vi "运维调试_氨氮.vi"() -> ()   [LabVIEW 2016, in "斯坦道氨氮.lvlib"]
uses:
  <vilib>/Utility/miscctls.llb/LVPointTypeDef.ctl
  <vilib>/Utility/config.llb/NI_LVConfig.lvlib
  <vilib>/ptbypt/NI_PtbyPt.lvlib
panel:
  in  "远程标样校准":enum16{"标液1", "标液2", "标液3", "标液4"}(ring)
  in  "远程校准量程":enum16{"低量程", "高量程"}(ring)
  in  "曲线模型 2":cluster{"X^2":dbl, "X":dbl, "B":dbl, "r^2":dbl}(xcontrol)
  out "固件版本号":string
  in  "定时设置":cluster{"启动":bool, "控制命令":T1, "测量参数":T2}(xcontrol)
  out "模块版本号":string
  in  "校准按钮":T3
  out "单位:":T4(ring)
  out "运行状态":T5 {"数据时间:" format="%<%y/%m/%d %H:%M:%S>T"; "仪器时间:" format="%<%y/%m/%d %H:%M:%S>T"}
  out "二级权限":bool
  out "一级权限":bool
  out "输入密码":u32
  out "布尔":bool
  in  "仪器参数设置":bool
  in  "流程固件":bool
  in  "量程参数读取写入":T6
  in  "模块启用":bool
  in  "串口设置":bool
  in  "公式一键写入":bool
  in  "流程路径":path=path "C:/Users/STD/Documents/斯坦道流程文件/流程.xml"
  in  "曲线模型":cluster{"X^2":dbl, "X":dbl, "B":dbl, "r^2":dbl}(xcontrol)
  out "字符串":string
  in  "质控参数设置":bool
  out "温度2":sgl
  out "温度1":sgl
  out "ADC":sgl
  in  "数组":string[](array[string])
  in  "量程切换阈值写入":bool
  in  "量程切换阈值读取":bool
  in  "参数下拉列表":enum16{"总磷", "总氮", "氨氮"}(ring)=enum."氨氮"
  in  "量程下拉列表":enum16{"低量程", "高量程"}(ring)
  in  "测量模式下拉列表":enum16{"水样测量", "零点核查", "跨度核查", "标样核查", "加标回收"}(ring)
  in  "公式":cluster{"X^2":dbl, "X":dbl, "b":dbl}
  in  "写公式":bool
  in  "读公式":bool
  in  "返回":bool
  in  "设置":bool
  out "集成报警信息":string
  in  "停止":bool
  in  "手动启动":bool
  in  "单步测试":bool
  out "F3":sgl format="%#.6f"
  out "F2":sgl format="%#.6f"
  out "F1":sgl format="%#.6f"
  out "F0":sgl format="%#.6f"
  out "多列列表框":i32(listbox)
  # "参数设置"
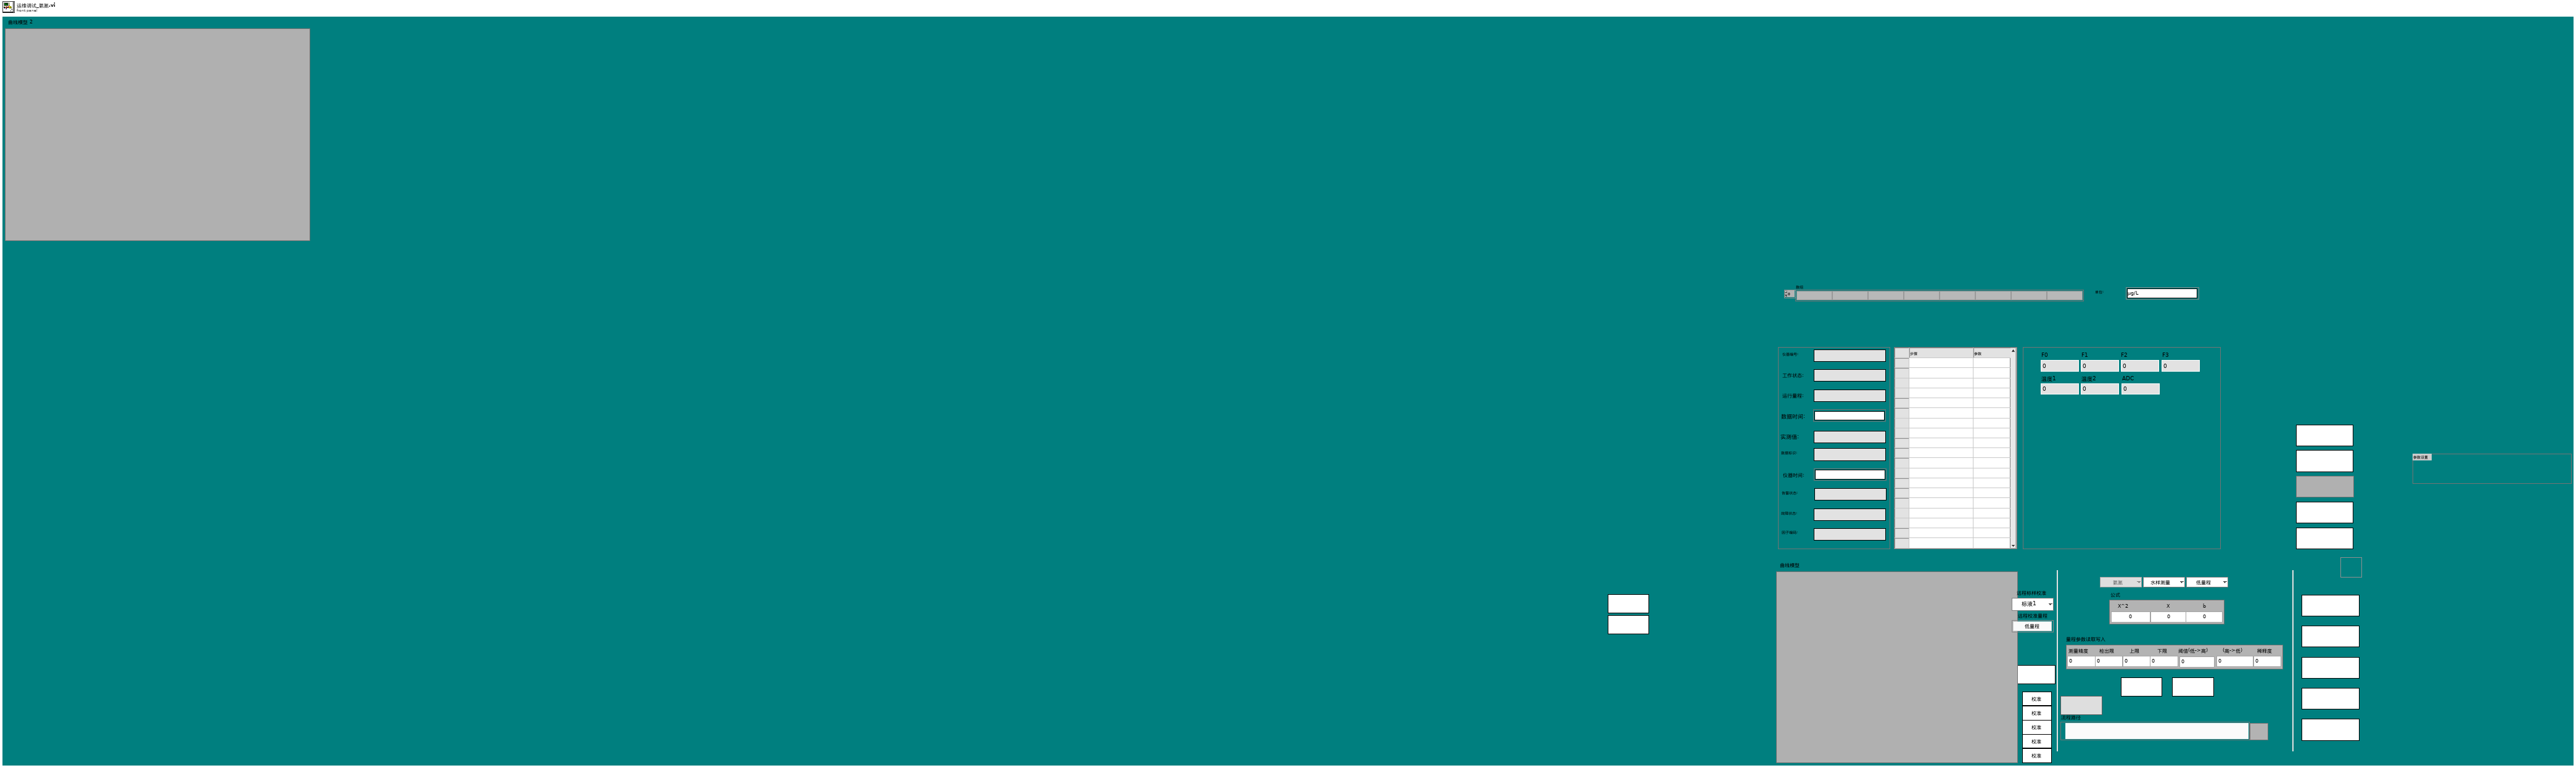
[diagram p1: front panel]
types:
  T1 = typedef "定时设置.xctl/国标控制命令.ctl" = enum16{"启动测量", "标样核查", "零点核查", "跨度核查", "空白测试", "平行样测试", "加标回收", "空白校准", "标样校准", "初始化（清洗）", "停止测试", "仪器重启", "校时", "模式设置", "测量间隔设置"}
  T2 = typedef "定时设置.xctl/测量参数.ctl" = u16
  T3 = cluster{"校准1":bool, "校准2":bool, "校准3":bool, "校准4":bool, "校准5":bool}
  T4 = enum16{"μg/L", "mg/L", "ppm", "mg/m3", "cm", "ppb", "μg/m3", "%", "nmol/mol", "μmol/mol", "MPN/L", "MPN/100ml", "ng/m3", "NTU", "无量纲", "mS/cm", "μS/cm", "℃", "mV", "cells/mL"}
  T5 = cluster{"仪器编号:":string, "工作状态:":string, "运行量程: ":string, "数据时间:":timestamp, "实测值:":string, "数据标识: ":string, "仪器时间:":timestamp, "告警状态: ":string, "故障状态:  ":string, "因子编码:":string}
  T6 = cluster{"测量精度":dbl, "检出限":dbl, "上限":dbl, "下限":dbl, "阈值(低->高)":dbl, "(高->低)":dbl, "稀释度":dbl}
  T7 = typedef "LVPointTypeDef.ctl" = cluster{"Horizontal":i16, "Vertical":i16}
  T8 = cluster{"时间源选择":enum16{"系统时间源", "仪器时间源"}, "外部时间源":timestamp}
  T9 = enum16{"空闲", "水样测试", "标样核查", "零点核查", "跨度核查", "空白测试", "平行样测试", "加标回收", "空白校准", "标样校准", "初始化（清洗）"}
  T10 = cluster{"系统时间":timestamp, "工作状态":enum16{"空闲", "水样测试", "标样核查", "零点核查", "跨度核查", "空白测试", "平行样测试", "加标回收", "空白校准", "标样校准", "初始化（清洗）"}, "测量模式":enum16{"待机", "连续模式", "周期模式", "定点模式", "受控模式", "手动模式"}, "告警代码":u16, "故障代码":u16, "日志代码":u16, "软件版本":u16, "F0":sgl, "F1":sgl, "F2":sgl, "F3":sgl, "T":sgl, "H":sgl, "id":u16, "flowid":u16, "量程":u16, "总磷控温温度1":sgl, "营养盐控温温度2":sgl, "ADC":sgl}
  T11 = enum32{"Bad", "Idle", "Run top level", "Running"}
  T12 = enum8{"Enabled", "Disabled", "Disabled and Grayed Out"}
  T13 = cluster{"运行模式":enum16{"维护模式", "常规模式", "应急模式", "质控模式"}, "质控频次":enum16{"关闭", "每天", "星期一", "星期二", "星期三", "星期四", "星期五", "星期六", "星期日"}, "空白核查时间":u16, "跨度核查时间":u16, "24H周期设置":bool[]}
  T14 = cluster{"因子编码":u32, "单位":u16, "标样参考值":sgl, "水样数据时间":timestamp, "水样实测值":sgl, "水样数据标识":string, "标样数据时间":timestamp, "标样实测值":sgl, "标样数据标识":string, "空白数据时间":timestamp, "空白实测值":sgl, "空白数据标识":string, "零点核查数据时间":timestamp, "零点核查实测值":sgl, "零点核查数据标识":string, "跨度核查数据时间":timestamp, "跨度核查实测值":sgl, "跨度核查数据标识":string, "加标回收数据时间":timestamp, "加标回收实测值":sgl, "加标回收数据标识":string, "平行样数据时间":timestamp, "平行样实测值":sgl, "平行样数据标识":string, "F0":sgl, "F1":sgl, "F2":sgl, "F3":sgl, "F4":sgl, "F5":sgl, "F6":sgl, "F7":sgl, "温度":sgl, "湿度":sgl, "X值":sgl, "fidrange":u16}
  T15 = cluster{"Major":u16, "Minor":u16, "Fix":u16, "Build":u16}
  T16 = typedef "NI_LVConfig.lvlib/Config Data RefNum.ctl" = refnum<k1>
  T17 = cluster{"时间标识":timestamp, "设备":string, "日志信息":string, "备注":string}
  T18 = cluster{"参数":string, "报警内容":string, "报警分析":string}
  T19 = cluster{"参数下拉列表":enum16{"总磷", "总氮", "氨氮"}, "测量模式下拉列表":enum16{"水样测量", "零点核查", "跨度核查", "标样核查", "加标回收"}, "量程下拉列表":enum16{"低量程", "高量程"}}
  T20 = cluster{"启动模式":enum16{"跨度核查", "水样测量", "空白核查", "标样核查", "加标回收"}, "启动参数":u16, "量程":enum16{"低量程", "高量程"}}
  T21 = cluster{"时间标识":timestamp, "设备":string, "日志信息":string, "流程参数":string}
  T22 = typedef "LVRowAndColumnUnsignedTypeDef.ctl" = cluster{"Row":u32, "Column":u32}
  T23 = cluster{"站号":u16, "量程切换":enum32{"H", "L", "AUTO"}, "控制命令":enum16{"启动测量", "标样核查", "零点核查", "跨度核查", "空白测试", "平行样测试", "加标回收", "空白校准", "标样校准", "初始化（清洗）", "停止测试", "仪器重启", "校时", "模式设置", "测量间隔设置"}, "模式设置":enum16{"待机", "连续模式", "周期模式", "定点模式", "受控模式", "手动模式"}, "测量间隔":u16}
  T24 = cluster{"标液浓度1":dbl, "标液浓度2":dbl, "标液浓度3":dbl, "标液浓度4":dbl, "标液浓度5":dbl}
  T25 = cluster{"水样测试量程模式":enum16{"H", "L", "AUTO"}, "空白核查量程模式":enum16{"H", "L", "AUTO"}, "跨度核查量程模式":enum16{"H", "L", "AUTO"}, "加标回收量程模式":enum16{"H", "L", "AUTO"}}
  T26 = cluster{"跨度值":dbl, "零点标准液浓度":dbl, "跨度标准液浓度":dbl, "标准液标准浓度":dbl}
  T27 = cluster{"确定":bool, "跨度值":dbl, "零点标准液浓度":dbl, "跨度标准液浓度":dbl, "标准液标准浓度":dbl}
  T28 = cluster{"测量量程":dbl, "测量精度":dbl, "测量间隔":dbl, "消解温度":dbl, "消解时长":dbl, "空白校准时间":timestamp, "曲线截距":dbl, "曲线斜率":dbl, "测量检出限":dbl, "测量信号值":dbl, "线性相关系数":dbl, "二次多项式系数":dbl, "标样校准时间":timestamp, "稀释倍数":dbl, "三项式系数":dbl, "空白标定系数":dbl, "量程系数":dbl, "F0/ORPA":dbl, "F1/ORPB":dbl, "F2/ORPK":dbl, "F3":dbl, "F4":dbl, "F5":dbl, "F6":dbl, "F7":dbl, "X0/滴定数":dbl, "量程":dbl}
  T29 = cluster{"确定":bool, "测量量程":dbl, "测量精度":dbl, "测量间隔":dbl, "消解温度":dbl, "消解时长":dbl, "空白校准时间":timestamp, "曲线截距":dbl, "曲线斜率":dbl, "测量检出限":dbl, "测量信号值":dbl, "线性相关系数":dbl, "二次多项式系数":dbl, "标样校准时间":timestamp, "稀释倍数":dbl, "三项式系数":dbl, "空白标定系数":dbl, "量程系数":dbl, "F0/ORPA":dbl, "F1/ORPB":dbl, "F2/ORPK":dbl, "F3":dbl, "F4":dbl, "F5":dbl, "F6":dbl, "F7":dbl, "X0/滴定数":dbl, "量程":dbl}
  T30 = cluster{"测量精度":u16, "检出限":dbl, "上限":dbl, "下限":dbl, "阈值（低->高）":dbl, "阈值（高->低）":dbl, "稀释度":dbl}
  T31 = enum16{"Left Button", "Center Button", "Right Button", "Window Close"}
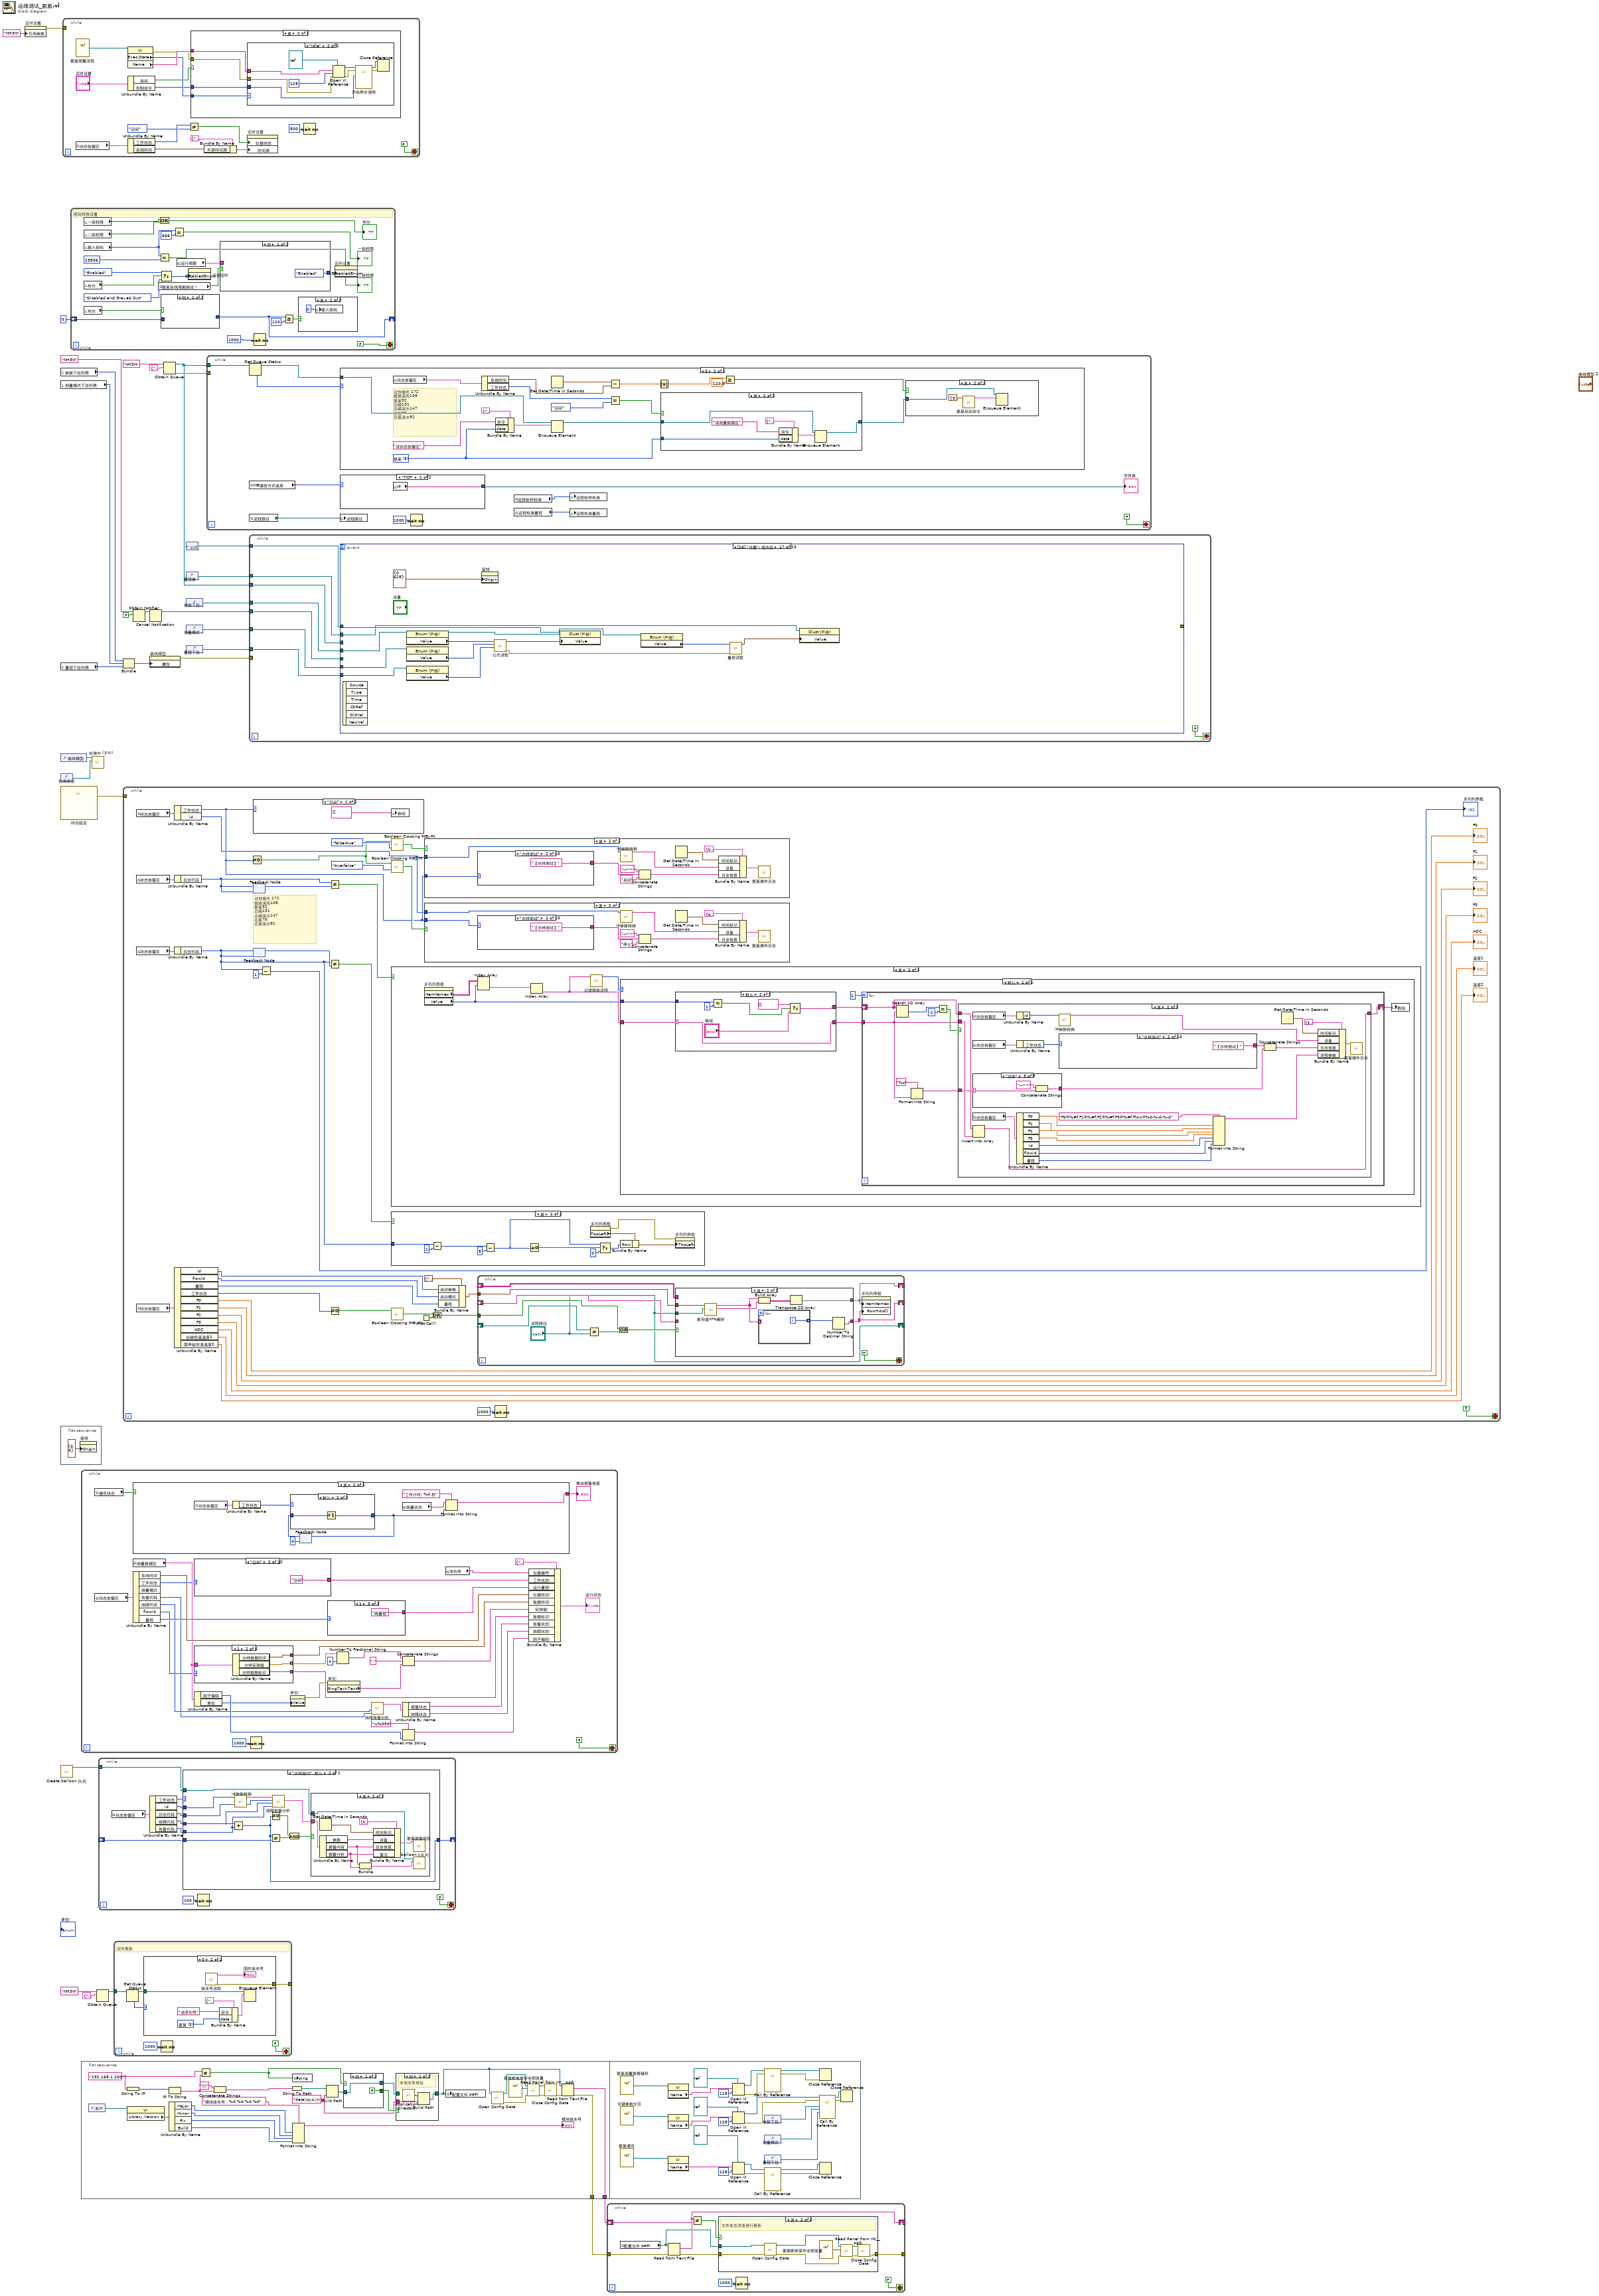
[diagram p0: block diagram]
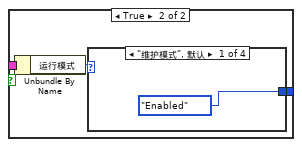
[diagram p5: hidden frame]
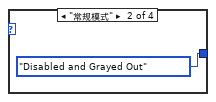
[diagram p6: hidden frame]
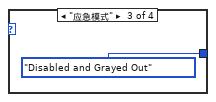
[diagram p7: hidden frame]
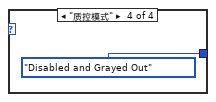
[diagram p8: hidden frame]
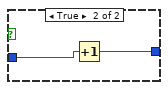
[diagram p10: hidden frame]
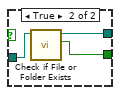
[diagram p11: hidden frame]
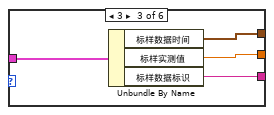
[diagram p15: hidden frame]
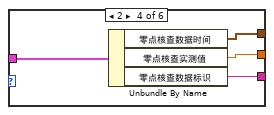
[diagram p16: hidden frame]
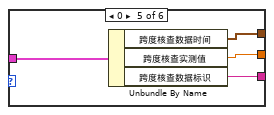
[diagram p17: hidden frame]
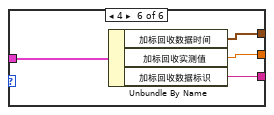
[diagram p18: hidden frame]
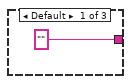
[diagram p19: hidden frame]
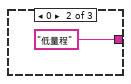
[diagram p20: hidden frame]
diagram:
  n1 = property on="定时设置" class="定时设置 (严格)"("引用参数"="NH3N") -> (error out=w2:errorcluster)  [unwired: 2 in, 1 out]
  n2 = local read "参数下拉列表"() -> (w11:enum16{"总磷", "总氮", "氨氮"})
  n3 = local read "测量模式下拉列表"() -> (w10:enum16{"水样测量", "零点核查", "跨度核查", "标样核查", "加标回收"})
  n4 = local read "量程下拉列表"() -> (w9:enum16{"低量程", "高量程"})
  n5 = control-ref of="曲线模型"() -> (w5:refnum<vi>)
  n6 = control-ref of="校准按钮"() -> (w4:refnum<vi>)
  n7 = call "时间延迟"() -> ("error out"=w22:errorcluster)  [unwired: 11 in]
  n8 = flat-sequence {
    frame #0 {
      n9 = property on="窗格" class="Pane"("Origin"=T7 {"Horizontal"=0, "Vertical"=0} ("原点")) -> ()  [unwired: 2 in, 2 out]
    }
  }
  n10 = call "Create balloon 队列.vi"() -> ("队列输出"=w3:refnum<queue>)  [unwired: 11 in]
  n11 = while {
    tunnel: w2 -> [_]
    stop <- FALSE stop-if-true
    n12 = vi-ref "氨氮测量流程.vi"() -> (w42:refnum<vi>)
    n13 = global read "VAR氨氮全局变量.vi" "状态告警区"() -> (w45:T10)
    n14 = property class="VI"(reference=w42) -> (error out=w39:errorcluster, "Exec.State"=w40:T11, "Name"=w41:string)  [unwired: 1 in, 1 out]
    n15 = Unbundle By Name("定时设置") -> ("启动"=w37:bool, "控制命令"=w36:T1)
    n16 = Unbundle By Name(w45) -> ("工作状态"=w44:T9, "系统时间"=w33:timestamp)
    n17 = Not Equal?(x=w44, y=T9."空闲") -> (x != y?=w35:bool)
    n18 = case shown="真" w37 {
      tunnel: w41 -> [_ w51]
      tunnel: w36 -> [_ w50]
      tunnel: w40 -> [_ w49]
      tunnel: w39 -> [_ w48]
      frame False {
      }
      frame True {
        n19 = case shown="\"Idle\"" w49 {
          tunnel: w51 -> [_ w56]
          tunnel: w50 -> [_ w54]
          tunnel: w48 -> [_ w52]
          frame "Bad", Default {
          }
          frame "Idle" {
            n20 = Open VI Reference(type specifier VI Refnum (for type only)=refnum<vi> refnum, vi path=w56, options=128 ("选项"), error in (no error)=w52) -> (vi reference=w57:refnum<vi>, error out=w58:errorcluster)  [unwired: 2 in]
            n21 = call-by-ref "开始异步调用"(reference=w57, error in=w58, "控制命令"=w54) -> (reference out=w59:refnum<vi>, error out=w60:errorcluster)  [unwired: 11 in]
            n22 = Close Reference(reference=w59, error in (no error)=w60) -> ()  [unwired: 1 out]
          }
        }
      }
    }
    n23 = Bundle By Name(cluster=T8 {"时间源选择"=enum."仪器时间源", "外部时间源"=timestamp(0 s since 1904-01-01)} ("时间源"), "外部时间源"=w33) -> (w32:T8)
    n24 = property on="定时设置" class="定时设置 (严格)"("仪器状态"=w35, "时间源"=w32) -> ()  [unwired: 2 in, 2 out]
    n25 = Wait (ms)(milliseconds to wait=u32 500 ("等待时间（毫秒）")) -> ()  [unwired: 1 out]
  }
  n26 = while {
    shift-right: [w66] -> _
    shift-left: u32 0 ("等待时间（毫秒）") -> [w67]
    stop <- FALSE stop-if-true
    # "密码权限设置"
    n27 = local read "一级权限"() -> (w75:bool)
    n28 = local read "二级权限"() -> (w76:bool)
    n29 = local read "输入密码"() -> (w79:u32)
    n30 = local read "布尔"() -> (w70:bool)
    n31 = local read "布尔"() -> (w68:bool)
    n32 = global read "氨氮断电保存全局变量.vi" "氨氮系统周期测试？"() -> (w61:bool)
    n33 = Or(x=w75, y=w76) -> (x .or. y?=→"布尔":bool)
    n34 = Equal?(x=w79, y=u32 23506) -> (x = y?=→"二级权限":bool)
    n35 = Select(t=T12."Enabled" ("禁用"), s=w70, f=T12."Disabled and Grayed Out") -> (s? t:f=w71:T12)
    n36 = case shown="假" w68 {
      tunnel: w67 -> [_ w93]
      tunnel: [_ w92] -> w66
      frame False {
      }
      frame True {
        n37 = Increment(x=w93) -> (x+1=w92:u32)
      }
    }
    n38 = Equal?(x=w79, y=u32 666) -> (x = y?=→"一级权限":bool)
    n39 = global read "氨氮断电保存全局变量.vi" "运行周期"() -> (w63:T13)
    n40 = property on="流程固件" class="Bool"("DisabledEnum"=w71) -> ()  [unwired: 2 in, 2 out]
    n41 = case shown="假" w61 {
      tunnel: w63 -> [_ w86]
      tunnel: [T12."Enabled" ("禁用") w84] -> w62
      frame False {
      }
      frame True {
        n42 = Unbundle By Name(w86) -> ("运行模式"=w85:enum16{"维护模式", "常规模式", "应急模式", "质控模式"})
        n43 = case shown="\"维护模式\", 默认" w85 {
          tunnel: [T12."Enabled" ("禁用") T12."Disabled and Grayed Out" ("禁用") T12."Disabled and Grayed Out" ("禁用") T12."Disabled and Grayed Out" ("禁用")] -> w84
          frame "维护模式", Default {
          }
          frame "常规模式" {
          }
          frame "应急模式" {
          }
          frame "质控模式" {
          }
        }
      }
    }
    n44 = Wait (ms)(milliseconds to wait=u32 1000 ("等待时间（毫秒）")) -> ()  [unwired: 1 out]
    n45 = Greater Or Equal?(x=w66, y=u32 120) -> (x >= y?=w64:bool)
    n46 = case shown="真" w64 {
      frame False {
      }
      frame True {
        n47 = local write "输入密码"(u32 0 ("输入密码")) -> ()
      }
    }
    n48 = property on="定时设置" class="定时设置 (严格)"("DisabledEnum"=w62) -> ()  [unwired: 2 in, 2 out]
  }
  n49 = while {
    stop <- FALSE stop-if-true
    n50 = global read "VAR氨氮全局变量.vi" "通讯状态"() -> (w124:bool)
    n51 = global read "VAR氨氮全局变量.vi" "状态告警区"() -> (w122:T10)
    n52 = case shown="真" w124 {
      tunnel: ["通讯异常" ("集成报警信息") w167] -> w123
      frame False {
      }
      frame True {
        n53 = global read "VAR氨氮全局变量.vi" "状态告警区"() -> (w173:T10)
        n54 = Unbundle By Name(w173) -> ("工作状态"=w172:T9)
        n55 = feedback #1(0) -> (w170:i32)
        n56 = case shown="默认" w172 {
          tunnel: w170 -> [_ w175]
          tunnel: [_ w174] -> w168
          frame "空闲" {
          }
          frame Default {
            n57 = Increment(x=w175) -> (x+1=w174:i32)
          }
        }
        n58 = feedback-in #1(w168) -> ()
        n59 = global read "VAR氨氮全局变量.vi" "测量状态"() -> (w166:string)
        n60 = Format Into String(format string="工作计时: %d 秒" ("格式字符串"), initial string=w166, w168) -> (resulting string=w167:string)  [unwired: 1 in, 1 out]
      }
    }
    "集成报警信息" <- w123
    n61 = global read "VAR氨氮全局变量.vi" "测量数据区"() -> (w114:T14)
    n62 = Unbundle By Name(w122) -> ("系统时间"=w120:timestamp, "工作状态"=w113:T9, "告警代码"=w94:u16, "故障代码"=w95:u16, "flowid"=w112:u16, "量程"=w118:u16)  [unwired: 1 out]
    n63 = case shown="\"空闲\"" w113 {
      selector: w113 -> [w150 _ _ _ _ _ _ _ _ _ _ _]
      tunnel: [w151 "空闲" ("工作状态") "水样测量" ("工作状态") "标样核查" ("工作状态") "零点核查" ("工作状态") "跨度核查" ("工作状态") "空白测试" ("工作状态") "平行样测试" ("工作状态") "加标回收" ("工作状态") "空白校准" ("工作状态") "标样校准" ("工作状态") "初始化" ("工作状态")] -> w119
      frame Default {
        n64 = Format Into String(format string="%d" ("格式字符串"), initial string="未知" ("工作状态"), w150) -> (resulting string=w151:string)  [unwired: 1 in, 1 out]
      }
      frame "空闲" {
      }
      frame "水样测试" {
      }
      frame "标样核查" {
      }
      frame "零点核查" {
      }
      frame "跨度核查" {
      }
      frame "空白测试" {
      }
      frame "平行样测试" {
      }
      frame "加标回收" {
      }
      frame "空白校准" {
      }
      frame "标样校准" {
      }
      frame "初始化（清洗）" {
      }
    }
    n65 = case shown="1" w112 {
      tunnel: [_ w130 w134 w138 w142 w146] -> w103
      tunnel: [_ w128 w133 w137 w141 w145] -> w108
      tunnel: [_ w127 w132 w136 w140 w144] -> w102
      tunnel: w114 -> [_ w129 w131 w135 w139 w143]
      frame Default {
      }
      frame 1 {
        n66 = Unbundle By Name(w129) -> ("水样数据时间"=w130:timestamp, "水样实测值"=w128:sgl, "水样数据标识"=w127:string)
      }
      frame 3 {
        n67 = Unbundle By Name(w131) -> ("标样数据时间"=w134:timestamp, "标样实测值"=w133:sgl, "标样数据标识"=w132:string)
      }
      frame 2 {
        n68 = Unbundle By Name(w135) -> ("零点核查数据时间"=w138:timestamp, "零点核查实测值"=w137:sgl, "零点核查数据标识"=w136:string)
      }
      frame 0 {
        n69 = Unbundle By Name(w139) -> ("跨度核查数据时间"=w142:timestamp, "跨度核查实测值"=w141:sgl, "跨度核查数据标识"=w140:string)
      }
      frame 4 {
        n70 = Unbundle By Name(w143) -> ("加标回收数据时间"=w146:timestamp, "加标回收实测值"=w145:sgl, "加标回收数据标识"=w144:string)
      }
    }
    n71 = Unbundle By Name(w114) -> ("因子编码"=w115:u32, "单位"=w109:u16)
    n72 = Wait (ms)(milliseconds to wait=u32 1000 ("等待时间（毫秒）")) -> ()  [unwired: 1 out]
    n73 = property on="单位:" class="Enum (严格)"("Value"=w109) -> (error out=w110:errorcluster)  [unwired: 2 in, 1 out]
    n74 = case shown="1" w118 {
      tunnel: ["" ("字符串") "低量程" ("字符串") "高量程" ("字符串")] -> w117
      frame Default {
      }
      frame 0 {
      }
      frame 1 {
      }
    }
    n75 = property on="单位:" class="Enum (严格)"(error in=w110) -> ("RingText.Text"=w99:string)  [unwired: 1 in, 2 out]
    n76 = Number To Fractional String(number=w108, precision (6)=i16 4 ("精度(6)")) -> (F-format string=w106:string)  [unwired: 2 in]
    n77 = call "故障告警分析.vi"("告警代码"=w94, "故障代码"=w95) -> ("简易报警状态"=w98:cluster{"故障状态":string, "报警状态":string})  [unwired: 8 in, 1 out]
    n78 = Concatenate Strings(w106, " " ("字符串"), w99) -> (w105:string)
    n79 = Unbundle By Name(w98) -> ("报警状态"=w97:string, "故障状态"=w96:string)
    n80 = Format Into String(format string="w%05d" ("格式字符串"), w115) -> (resulting string=w104:string)  [unwired: 2 in, 1 out]
    n81 = global read "VAR氨氮全局变量.vi" "序列号"() -> (w121:string)
    n82 = Bundle By Name(cluster=T5 {"仪器编号:"="", "工作状态:"="", "运行量程: "="", "数据时间:"=timestamp(0 s since 1904-01-01), "实测值:"="", "数据标识: "="", "仪器时间:"=timestamp(0 s since 1904-01-01), "告警状态: "="", "故障状态:  "="", "因子编码:"=""} ("运行状态"), "仪器编号:"=w121, "工作状态:"=w119, "运行量程:"=w117, "仪器时间:"=w120, "数据时间:"=w103, "实测值:"=w105, "数据标识:"=w102, "告警状态:"=w97, "故障状态:"=w96, "因子编码:"=w104) -> (→"运行状态":T5)
  }
  n83 = flat-sequence {
    tunnel: [w185] -> w7
    tunnel: [w184] -> w6
    frame #0 {
      w197 = "data\\sys.ini" ("名称或相对路径")
      w189 = "192.168.1.100" ("名称")
      n84 = control-ref of="本VI"() -> (w183:refnum<vi>)
      n85 = String To IP(1:w189) -> (0:w196:u32)
      n86 = property class="VI"(reference=w183) -> ("Library.Version"=w182:T15)  [unwired: 1 in, 2 out]
      n87 = IP To String(2:w196) -> (0:w193:string)  [unwired: 1 in]
      n88 = Unbundle By Name(w182) -> ("Major"=w180:u16, "Minor"=w179:u16, "Fix"=w178:u16, "Build"=w177:u16)
      n89 = Not Equal?(x=w189, y=w193) -> (x != y?=w198:bool)
      n90 = Concatenate Strings("\\\\" ("字符串"), w193) -> (w194:string)
      n91 = String To Path(string=w194) -> (path=w188:path)
      n92 = global write "VAR氨氮全局变量.vi" "ping"(w198) -> ()
      n93 = Format Into String(format string="模块版本号：%d.%d.%d.%d" ("格式字符串"), w180, w179, w178, w177) -> (resulting string=→"模块版本号":string)  [unwired: 2 in, 1 out]
      n94 = Build Path(base path=w188, name or relative path=w197) -> (appended path=w192:path)
      n95 = case shown="假" w198 {
        tunnel: w192 -> [w204 w208]
        tunnel: [w204 w207] -> w191
        tunnel: [FALSE w206] -> w190
        frame False {
        }
        frame True {
          n96 = call <vilib>:"Check if File or Folder Exists.vi"("path"=w208) -> ("file or folder exists?"=w206:bool, "dup path"=w207:path)  [unwired: 8 in, 1 out]
        }
      }
      n97 = case shown="假" w190 {
        tunnel: w191 -> [_ w212]
        tunnel: [w210 w212] -> w187
        tunnel: w197 -> [w209 _]
        frame False {
          # "本地文件地址"
          n98 = call <vilib>:"Application Directory.vi"() -> ("Application Directory"=w211:path)
          n99 = Build Path(base path=w211, name or relative path=w209) -> (appended path=w210:path)
        }
        frame True {
          # "网络共享地址"
        }
      }
      n100 = global write "VAR氨氮全局变量.vi" "配置文件 path"(w187) -> ()
      n101 = call <vilib>:"Open Config Data.vi"("configuration file path"=w187) -> ("error out"=w200:errorcluster, "refnum"=w203:T16)  [unwired: 8 in, 1 out]
      n102 = vi-ref "氨氮断电保存全局变量.vi"() -> (w202:refnum<vi>)
      n103 = call <userlib>:"Read Panel from INI__ogtk.vi"("error in (no error)"=w200, "VI ref"=w202, "refnum"=w203) -> ("error out"=w199:errorcluster, "refnum out"=w201:T16)  [unwired: 7 in]
      n104 = call <vilib>:"Close Config Data.vi"("error in (no error)"=w199, "refnum"=w201) -> ("error out"=w186:errorcluster)  [unwired: 8 in, 1 out]
      n105 = Read from Text File(file (use dialog)=w187, error in=w186) -> (text=w184:string, error out=w185:errorcluster)  [unwired: 2 in, 2 out]
    }
    frame #1 {
      n106 = vi-ref "氨氮测量数据储存.vi"() -> (w231:refnum<vi>)
      n107 = vi-ref "关键参数交互.vi"() -> (w216:refnum<vi>)
      n108 = vi-ref "氨氮通讯.vi"() -> (w239:refnum<vi>)
      n109 = property class="VI"(reference=w231) -> ("Name"=w224:string)  [unwired: 1 in, 2 out]
      n110 = property class="VI"(reference=w216) -> ("Name"=w223:string)  [unwired: 1 in, 2 out]
      n111 = property class="VI"(reference=w239) -> ("Name"=w238:string)  [unwired: 1 in, 2 out]
      n112 = Open VI Reference(type specifier VI Refnum (for type only)=refnum<vi> refnum, vi path=w224, options=128 ("选项")) -> (vi reference=w226:refnum<vi>, error out=w228:errorcluster)  [unwired: 3 in]
      n113 = Open VI Reference(type specifier VI Refnum (for type only)=refnum<vi> refnum, vi path=w223, options=128 ("选项")) -> (vi reference=w221:refnum<vi>, error out=w219:errorcluster)  [unwired: 3 in]
      n114 = Open VI Reference(type specifier VI Refnum (for type only)=refnum<vi> refnum, vi path=w238, options=128 ("选项")) -> (vi reference=w236:refnum<vi>, error out=w234:errorcluster)  [unwired: 3 in]
      n115 = call-by-ref "?"(reference=w226, error in=w228) -> (reference out=w230:refnum<vi>, error out=w229:errorcluster)  [unwired: 12 in]
      n116 = control-ref of="参数下拉列表"() -> (w215:refnum<vi>)
      n117 = control-ref of="测量模式下拉列表"() -> (w214:refnum<vi>)
      n118 = control-ref of="量程下拉列表"() -> (w213:refnum<vi>)
      n119 = call-by-ref "?"(reference=w236, error in=w234) -> (reference out=w232:refnum<vi>, error out=w233:errorcluster)  [unwired: 12 in]
      n120 = Close Reference(reference=w230, error in (no error)=w229) -> ()  [unwired: 1 out]
      n121 = call-by-ref "?"(reference=w221, error in=w219, "量程下拉列表"=w213, "测量模式下拉列表"=w214, "参数下拉列表"=w215) -> (reference out=w217:refnum<vi>, error out=w218:errorcluster)  [unwired: 9 in]
      n122 = Close Reference(reference=w232, error in (no error)=w233) -> ()  [unwired: 1 out]
      n123 = Close Reference(reference=w217, error in (no error)=w218) -> ()  [unwired: 1 out]
    }
  }
  n124 = call "校准中 (子VI).vi"("曲线模型"=w5, "校准按钮"=w4) -> ()  [unwired: 9 in]
  n125 = Obtain Queue(name (unnamed)="NH3N" ("名称（未命名）"), element data type=cluster{"命令":string, "data":variant} {"命令"="", "data"=variant}) -> (queue out=w19:refnum<queue>)  [unwired: 3 in, 2 out]
  n126 = while {
    tunnel: w3 -> [w245]
    shift-right: [w241] -> _
    shift-left: _ -> [w242]
    stop <- FALSE stop-if-true
    n127 = global read "VAR氨氮全局变量.vi" "状态告警区"() -> (w249:T10)
    n128 = Unbundle By Name(w249) -> ("工作状态"=w240:T9, "id"=w247:u16, "日志代码"=w246:u16, "故障代码"=w244:u16, "告警代码"=w243:u16)
    n129 = case shown="\"水样测试\", 默认" w240 {
      tunnel: w247 -> [_ w263]
      tunnel: w246 -> [_ w262]
      tunnel: w245 -> [_ w259]
      tunnel: w244 -> [_ w258]
      tunnel: w243 -> [_ w257]
      tunnel: w242 -> [w251 w256]
      tunnel: [w251 w255] -> w241
      frame "空闲" {
      }
      frame "水样测试", Default {
        n130 = Add(x=w258, y=w257) -> (x+y=w255:u16)
        n131 = call "id参数转换.vi"("id"=w263) -> ("table输出"=w260:string)  [unwired: 10 in]
        n132 = Not Equal To 0?(x=w255) -> (x != 0?=w254:bool)
        n133 = Not Equal?(x=w255, y=w256) -> (x != y?=w253:bool)
        n134 = call "故障告警分析.vi"("告警代码"=w257, "故障代码"=w258, "运行步序"=w262, "参数"=w260) -> ("报警内容"=w261:T18)  [unwired: 6 in, 1 out]
        n135 = And(x=w254, y=w253) -> (x .and. y?=w252:bool)
        n136 = case shown="真" w252 {
          tunnel: w261 -> [_ w272]
          tunnel: w259 -> [_ w271]
          frame False {
          }
          frame True {
            n137 = Get Date/Time In Seconds() -> (seconds since 1Jan1904=w270:timestamp)
            n138 = Unbundle By Name(w272) -> ("参数"=w267:string, "报警内容"=w266:string, "报警分析"=w265:string)
            n139 = Bundle("报警内容"=w266, "报警分析"=w265) -> (w264:cluster{"报警内容":string, "报警分析":string})  [unwired: 1 in]
            n140 = Bundle By Name(cluster=T17 {"时间标识"=timestamp(0 s since 1904-01-01), "设备"="", "日志信息"="", "备注"=""} ("data in"), "时间标识"=w270, "设备"=w267, "日志信息"=w266, "备注"=w265) -> (w269:T17)
            n141 = call "氨氮报警信息.vi"("data in"=w269) -> ()  [unwired: 10 in, 1 out]
            n142 = call "balloon入队列.vi"("报警内容"=w264, "队列"=w271) -> ()  [unwired: 9 in, 1 out]
          }
        }
      }
    }
    n143 = Wait (ms)(milliseconds to wait=u32 100) -> ()  [unwired: 1 out]
  }
  n144 = while {
    tunnel: w19 -> [w277]
    tunnel: [w275] -> _
    stop <- FALSE stop-if-true
    # "定时更新"
    n145 = Get Queue Status(queue=w277) -> (queue out=w274:refnum<queue>, # elements in queue=w273:i32)  [unwired: 2 in, 6 out]
    n146 = case shown="0" w273 {
      tunnel: [_ w281] -> w275
      tunnel: w274 -> [_ w280]
      frame Default {
      }
      frame 0 {
        w283 = u16 3 items=["总磷"=1, "氨氮"=3] ("站号")
        n147 = call "版本号读取.vi"() -> ("error out"=w281:errorcluster, "固件版本号"=→"固件版本号":string)  [unwired: 10 in]
        n148 = Bundle By Name(cluster=cluster{"命令":string, "data":variant} {"命令"="", "data"=variant} ("元素"), "命令"="读序列号", "data"=w283) -> (w282:cluster{"命令":string, "data":variant})
        n149 = Enqueue Element(queue=w280, element=w282) -> ()  [unwired: 2 in, 3 out]
      }
    }
    n150 = Wait (ms)(milliseconds to wait=u32 1000 ("等待时间（毫秒）")) -> ()  [unwired: 1 out]
  }
  n151 = Bundle("参数下拉列表"=w11, "测量模式下拉列表"=w10, "量程下拉列表"=w9) -> (w12:T19)  [unwired: 1 in]
  n152 = while {
    tunnel: w22 -> [_]
    stop <- FALSE stop-if-true
    # "试剂填充 172 \n管路清洗108\n氨氮92\n总磷131\n总磷海水147\n总氮76\n总氮海水92"
    n153 = global read "VAR氨氮全局变量.vi" "状态告警区"() -> (w306:T10)
    n154 = global read "VAR氨氮全局变量.vi" "状态告警区"() -> (w304:T10)
    n155 = global read "VAR氨氮全局变量.vi" "状态告警区"() -> (w308:T10)
    n156 = global read "VAR氨氮全局变量.vi" "状态告警区"() -> (w316:T10)
    n157 = Unbundle By Name(w306) -> ("工作状态"=w287:T9, "id"=w286:u16)
    n158 = Unbundle By Name(w304) -> ("日志代码"=w303:u16)
    n159 = Unbundle By Name(w308) -> ("日志代码"=w300:u16)
    n160 = Unbundle By Name(w316) -> ("id"=w313:u16, "flowid"=w315:u16, "量程"=w314:u16, "工作状态"=w294:T9, "F0"=→"F0":sgl, "F1"=→"F1":sgl, "F2"=→"F2":sgl, "F3"=→"F3":sgl, "ADC"=→"ADC":sgl, "总磷控温温度1"=→"温度1":sgl, "营养盐控温温度2"=→"温度2":sgl)
    n161 = Not Equal To 0?(x=w287) -> (x != 0?=w289:bool)
    n162 = case shown="\"空闲\"" w287 {
      frame "空闲" {
        n163 = local write "数组"(string[] [] ("数组")) -> ()
      }
      frame "水样测试", Default {
      }
    }
    n164 = feedback #2(w303) -> (w305:u16)
    n165 = feedback-in #2(w303) -> ()
    n166 = feedback-in #3(w300) -> ()
    n167 = feedback #3(w300) -> (w321:u16)
    n168 = Subtract(x=w300, y=1) -> (x-y=→"多列列表框":i32)
    n169 = Not Equal?(x=w303, y=w305) -> (x != y?=w302:bool)
    n170 = Not Equal?(x=w300, y=w321) -> (x != y?=w320:bool)
    n171 = Not Equal To 0?(x=w294) -> (x != 0?=w318:bool)
    n172 = call <vilib>:"Boolean Crossing PtByPt.vi"("direction"=enum16{"either", "false-true", "true-false"}."false-true", "input"=w289) -> ("crossing"=w291:bool)  [unwired: 1 in]
    n173 = call <vilib>:"Boolean Crossing PtByPt.vi"("direction"=enum16{"either", "false-true", "true-false"}."true-false", "input"=w289) -> ("crossing"=w288:bool)  [unwired: 1 in]
    n174 = case shown="真" w302 {
      frame False {
      }
      frame True {
        n175 = property on="多列列表框" class="MCListbox (严格)"() -> ("ItemNames"=w367:string[][], "Value"=w363:i32)  [unwired: 2 in, 2 out]
        n176 = Index Array(array=w367, index (row)=w363) -> (element=w366:string[])  [unwired: 1 in]
        n177 = Index Array(array=w366) -> (element=w365:string)  [unwired: 1 in]
        n178 = call "过滤筛选流程.vi"("字符串"=w365) -> ("匹配后偏移量"=w364:i32)  [unwired: 10 in]
        n179 = case shown="默认" w364 {
          tunnel: w365 -> [w369 _]
          tunnel: w363 -> [w368 _]
          frame Default {
            n180 = case shown="默认" w369 {
              selector: w369 -> [w375 w382]
              tunnel: [w375 w382] -> w371
              tunnel: [string[] [] ("数组") w377] -> w370
              tunnel: w368 -> [_ w381]
              frame "读数" {
              }
              frame Default {
                n181 = Equal?(x=w381, y=1) -> (x = y?=w379:bool)
                n182 = Select(t=string[] [], s=w379, f="数组") -> (s? t:f=w377:string[])
              }
            }
            n183 = for {
              N: 1 -> [_]
              tunnel: w371 -> [w384]
              shift-right: [w383] -> w372
              shift-left: w370 -> [w385]
              n184 = Search 1D Array(1D array=w385, element=w384) -> (index of element=w388:i32)  [unwired: 1 in]
              n185 = Format Into String(format string="%s" ("格式字符串"), w384) -> (resulting string=w389:string)  [unwired: 2 in, 1 out]
              n186 = Equal?(x=w388, y=-1) -> (x = y?=w386:bool)
              n187 = case shown="真" w386 {
                tunnel: w389 -> [_ w399]
                tunnel: w385 -> [w391 w403]
                tunnel: w384 -> [_ w402]
                tunnel: [w391 w401] -> w383
                frame False {
                }
                frame True {
                  n188 = global read "VAR氨氮全局变量.vi" "状态告警区"() -> (w416:T10)
                  n189 = global read "VAR氨氮全局变量.vi" "状态告警区"() -> (w398:T10)
                  n190 = case shown="\"结束\"" w399 {
                    selector: w399 -> [w426 w429 w432]
                    tunnel: [w426 w428 w431] -> w395
                    frame Default {
                    }
                    frame "初始化" {
                      n191 = Concatenate Strings("-->>" ("字符串"), w429) -> (w428:string)
                    }
                    frame "结束" {
                      n192 = Concatenate Strings("-->>" ("字符串"), w432) -> (w431:string)
                    }
                  }
                  n193 = global read "VAR氨氮全局变量.vi" "状态告警区"() -> (w413:T10)
                  n194 = Insert Into Array(array=w403, new element=w402) -> (w401:string[])  [unwired: 1 in]
                  n195 = Unbundle By Name(w416) -> ("id"=w393:u16)
                  n196 = Unbundle By Name(w398) -> ("工作状态"=w397:T9)
                  n197 = Unbundle By Name(w413) -> ("F0"=w410:sgl, "F1"=w409:sgl, "F2"=w408:sgl, "F3"=w407:sgl, "id"=w406:u16, "flowid"=w405:u16, "量程"=w404:u16)
                  n198 = call "id参数转换.vi"("id"=w393) -> ("table输出"=w392:string)  [unwired: 10 in]
                  n199 = case shown="\"水样测试\"" w397 {
                    tunnel: [_ "【水样测试】" ("字符串") "【标样核查】" ("字符串") "【零点核查】" ("字符串") "【跨度核查】" ("字符串") "【空白测试】" ("字符串") "【平行样测试】" ("字符串") "【加标回收】" ("字符串") "【空白校准】" ("字符串") "【标样校准】" ("字符串")] -> w396
                    frame "空闲", Default {
                    }
                    frame "水样测试" {
                    }
                    frame "标样核查" {
                    }
                    frame "零点核查" {
                    }
                    frame "跨度核查" {
                    }
                    frame "空白测试" {
                    }
                    frame "平行样测试" {
                    }
                    frame "加标回收" {
                    }
                    frame "空白校准" {
                    }
                    frame "标样校准" {
                    }
                  }
                  n200 = Format Into String(format string="F0=%#f,F1=%#f,F2=%#f,F3=%#f,Flow=%d-%-d-%-d" ("格式字符串"), w410, w409, w408, w407, w406, w405, w404) -> (resulting string=w411:string)  [unwired: 2 in, 1 out]
                  n201 = Concatenate Strings(w396, w395) -> (w394:string)
                  n202 = Get Date/Time In Seconds() -> (seconds since 1Jan1904=w414:timestamp)
                  n203 = Bundle By Name(cluster=T21 {"时间标识"=timestamp(0 s since 1904-01-01), "设备"="", "日志信息"="", "流程参数"=""} ("data in"), "时间标识"=w414, "设备"=w392, "日志信息"=w394, "流程参数"=w411) -> (w415:T21)
                  n204 = call "氨氮操作日志.vi"("data in"=w415) -> ()  [unwired: 11 in]
                }
              }
            }
            n205 = local write "数组"(w372) -> ()
          }
          frame -1 {
          }
        }
      }
    }
    n206 = case shown="真" w320 {
      tunnel: w300 -> [_ w457]
      frame False {
      }
      frame True {
        n207 = Subtract(x=w457, y=1) -> (x-y=w455:i32)
        n208 = Subtract(x=w455, y=5) -> (x-y=w459:i32)
        n209 = Greater Or Equal To 0?(x=w459) -> (x >= 0?=w458:bool)
        n210 = property on="多列列表框" class="MCListbox (严格)"() -> (error out=w463:errorcluster, "TopLeft"=w464:T22)  [unwired: 2 in, 1 out]
        n211 = Select(t=w459, s=w458, f=0) -> (s? t:f=w460:i32)
        n212 = Bundle By Name(cluster=w464, "Row"=w460) -> (w465:T22)
        n213 = property on="多列列表框" class="MCListbox (严格)"(error in=w463, "TopLeft"=w465) -> ()  [unwired: 1 in, 2 out]
      }
    }
    n214 = call <vilib>:"Boolean Crossing PtByPt.vi"("input"=w318) -> ("crossing"=w293:bool)  [unwired: 2 in]
    n215 = First Call?() -> (First Call?: T/F=w319:bool)
    n216 = case shown="真" w291 {
      tunnel: w286 -> [_ w344]
      tunnel: w287 -> [_ w349]
      frame False {
      }
      frame True {
        n217 = case shown="\"水样测试\"" w349 {
          tunnel: [_ "【水样测试】" ("字符串") "【标样核查】" ("字符串") "【零点核查】" ("字符串") "【跨度核查】" ("字符串") "【空白测试】" ("字符串") "【平行样测试】" ("字符串") "【加标回收】" ("字符串") "【空白校准】" ("字符串") "【标样校准】" ("字符串")] -> w348
          frame "空闲", Default {
          }
          frame "水样测试" {
          }
          frame "标样核查" {
          }
          frame "零点核查" {
          }
          frame "跨度核查" {
          }
          frame "空白测试" {
          }
          frame "平行样测试" {
          }
          frame "加标回收" {
          }
          frame "空白校准" {
          }
          frame "标样校准" {
          }
        }
        n218 = call "id参数转换.vi"("id"=w344) -> ("table输出"=w343:string)  [unwired: 10 in]
        n219 = Concatenate Strings("-->>" ("字符串"), w348, "启动" ("字符串")) -> (w347:string)
        n220 = Get Date/Time In Seconds() -> (seconds since 1Jan1904=w351:timestamp)
        n221 = Bundle By Name(cluster=T21 {"时间标识"=timestamp(0 s since 1904-01-01), "设备"="", "日志信息"="", "流程参数"=""} ("data in"), "时间标识"=w351, "设备"=w343, "日志信息"=w347) -> (w350:T21)
        n222 = call "氨氮操作日志.vi"("data in"=w350) -> ()  [unwired: 11 in]
      }
    }
    n223 = case shown="真" w288 {
      tunnel: w286 -> [_ w325]
      tunnel: w287 -> [_ w330]
      frame False {
      }
      frame True {
        n224 = case shown="\"水样测试\"" w330 {
          tunnel: [_ "【水样测试】" ("字符串") "【标样核查】" ("字符串") "【零点核查】" ("字符串") "【跨度核查】" ("字符串") "【空白测试】" ("字符串") "【平行样测试】" ("字符串") "【加标回收】" ("字符串") "【空白校准】" ("字符串") "【标样校准】" ("字符串")] -> w329
          frame "空闲", Default {
          }
          frame "水样测试" {
          }
          frame "标样核查" {
          }
          frame "零点核查" {
          }
          frame "跨度核查" {
          }
          frame "空白测试" {
          }
          frame "平行样测试" {
          }
          frame "加标回收" {
          }
          frame "空白校准" {
          }
          frame "标样校准" {
          }
        }
        n225 = call "id参数转换.vi"("id"=w325) -> ("table输出"=w324:string)  [unwired: 10 in]
        n226 = Concatenate Strings("-->>" ("字符串"), w329, "停止" ("字符串")) -> (w328:string)
        n227 = Get Date/Time In Seconds() -> (seconds since 1Jan1904=w332:timestamp)
        n228 = Bundle By Name(cluster=T21 {"时间标识"=timestamp(0 s since 1904-01-01), "设备"="", "日志信息"="", "流程参数"=""} ("data in"), "时间标识"=w332, "设备"=w324, "日志信息"=w328) -> (w331:T21)
        n229 = call "氨氮操作日志.vi"("data in"=w331) -> ()  [unwired: 11 in]
      }
    }
    n230 = Or(x=w293, y=w319) -> (x .or. y?=w317:bool)
    n231 = Bundle By Name(cluster=T20 {"启动模式"=enum."跨度核查", "启动参数"=1, "量程"=enum."低量程"} ("参数簇"), "启动参数"=w313, "启动模式"=w315, "量程"=w314) -> (w307:T20)
    n232 = while {
      tunnel: w317 -> [w443]
      tunnel: w307 -> [w442]
      shift-right: [w437] -> _
      shift-left: _ -> [w439]
      shift-right: [w438] -> _
      shift-left: _ -> [w440]
      shift-right: ["流程路径"] -> _
      shift-left: _ -> [w436]
      stop <- TRUE stop-if-true
      n233 = Not Equal?(x=w436, y="流程路径") -> (x != y?=w434:bool)
      n234 = Or(x=w443, y=w434) -> (x .or. y?=w435:bool)
      n235 = case shown="真" w435 {
        tunnel: [w445 w453] -> w438
        tunnel: [w444 w452] -> w437
        tunnel: w442 -> [_ w447]
        tunnel: w440 -> [w445 _]
        tunnel: w439 -> [w444 _]
        tunnel: "流程路径" -> [_ w446]
        frame False {
        }
        frame True {
          n236 = call "斯坦道XML解析.vi"("添加的路径"=w446, "参数簇"=w447) -> ("步骤时间"=w448:string[], "步骤名"=w450:string[])  [unwired: 8 in]
          n237 = Build Array(w450, w448) -> (w449:string[][])
          n238 = for {
            tunnel: w450 -> [_] mode=indexing
            tunnel: [w454] -> w451 mode=indexing
            i -> [w454]
          }
          n239 = Transpose 2D Array(2D array=w449) -> (transposed array=w452:string[][])
          n240 = Number To Decimal String(number=w451) -> (decimal integer string=w453:string[])  [unwired: 1 in]
        }
      }
      n241 = property on="多列列表框" class="MCListbox (严格)"("ItemNames"=w437, "RowHdrs[]"=w438) -> ()  [unwired: 2 in, 2 out]
    }
    n242 = Wait (ms)(milliseconds to wait=u32 1000 ("等待时间（毫秒）")) -> ()  [unwired: 1 out]
  }
  n243 = Obtain Notifier(name (unnamed)="NH3N" ("名称（未命名）"), notification data type=FALSE) -> (notifier out=w15:refnum<notifier>)  [unwired: 2 in, 2 out]
  n244 = Cancel Notification(0:w15) -> (8:w14:refnum<notifier>)  [unwired: 1 in, 2 out]
  n245 = property on="曲线模型" class="曲线模型 (严格)"("属性"=w12) -> (error out=w18:errorcluster)  [unwired: 2 in, 1 out]
  n246 = Obtain Queue(name (unnamed)="NH3N" ("名称（未命名）"), element data type=cluster{"命令":string, "data":variant} {"命令"="", "data"=variant}) -> (queue out=w27:refnum<queue>, error out=w28:errorcluster)  [unwired: 3 in, 1 out]
  n247 = control-ref of="公式"() -> (w23:refnum<vi>)
  n248 = control-ref of="量程参数读取写入"() -> (w13:refnum<vi>)
  n249 = control-ref of="参数下拉列表"() -> (w25:refnum<vi>)
  n250 = control-ref of="测量模式下拉列表"() -> (w24:refnum<vi>)
  n251 = control-ref of="量程下拉列表"() -> (w26:refnum<vi>)
  n252 = while {
    tunnel: w27 -> [w473]
    tunnel: w28 -> [_]
    stop <- FALSE stop-if-true
    n253 = Get Queue Status(queue=w473) -> (queue out=w469:refnum<queue>, # elements in queue=w468:i32)  [unwired: 2 in, 6 out]
    n254 = global read "氨氮断电保存全局变量.vi" "MB通信方式选择"() -> (w470:enum16{"串口", "TCP"})
    n255 = global read "氨氮断电保存全局变量.vi" "流程路径"() -> (w472:path)
    n256 = case shown="0" w468 {
      tunnel: w469 -> [_ w479]
      frame Default {
      }
      frame 0 {
        w488 = u16 3 items=["总磷"=1, "氨氮"=3] ("站号")
        # "试剂填充 172 \n管路清洗108\n氨氮92\n总磷131\n总磷海水147\n总氮76\n总氮海水92"
        n257 = global read "VAR氨氮全局变量.vi" "状态告警区"() -> (w480:T10)
        n258 = Unbundle By Name(w480) -> ("系统时间"=w487:timestamp, "工作状态"=w478:T9)
        n259 = Bundle By Name(cluster=cluster{"命令":string, "data":variant} {"命令"="", "data"=variant} ("元素"), "命令"="读状态告警区", "data"=w488) -> (w491:cluster{"命令":string, "data":variant})
        n260 = Get Date/Time In Seconds() -> (seconds since 1Jan1904=w486:timestamp)
        n261 = Enqueue Element(queue=w479, element=w491) -> (queue out=w489:refnum<queue>)  [unwired: 2 in, 2 out]
        n262 = Subtract(x=w486, y=w487) -> (x-y=w485:dbl)
        n263 = Equal?(x=w478, y=T9."空闲") -> (x = y?=w476:bool)
        n264 = Absolute Value(x=w485) -> (abs(x)=w484:dbl)
        n265 = case shown="真" w476 {
          tunnel: w489 -> [w493 w496]
          tunnel: w488 -> [_ w495]
          tunnel: [w493 w494] -> w481
          frame False {
          }
          frame True {
            n266 = Bundle By Name(cluster=cluster{"命令":string, "data":variant} {"命令"="", "data"=variant} ("元素"), "命令"="读测量数据区", "data"=w495) -> (w498:cluster{"命令":string, "data":variant})
            n267 = Enqueue Element(queue=w496, element=w498) -> (queue out=w494:refnum<queue>)  [unwired: 2 in, 2 out]
          }
        }
        n268 = Greater Or Equal?(x=w484, y=120.0) -> (x >= y?=w482:bool)
        n269 = case shown="真" w482 {
          tunnel: w481 -> [_ w501]
          frame False {
          }
          frame True {
            n270 = call "氨氮启动命令.vi"("参数"=T23 {"站号"=3, "量程切换"=enum."AUTO", "控制命令"=enum."校时", "模式设置"=enum."待机", "测量间隔"=0}) -> ("启动命令"=w500:cluster{"命令":string, "data":variant})  [unwired: 10 in]
            n271 = Enqueue Element(queue=w501, element=w500) -> ()  [unwired: 2 in, 3 out]
          }
        }
      }
    }
    n272 = case shown="\"TCP\"" w470 {
      tunnel: [w503 w504] -> w471
      frame "串口", Default {
        n273 = global read "氨氮断电保存全局变量.vi" "VISA Resource"() -> (w503:refnum<visa-resource-name>)
      }
      frame "TCP" {
        n274 = global read "氨氮断电保存全局变量.vi" "IP"() -> (w504:string)
      }
    }
    "字符串" <- w471
    n275 = local write "流程路径"(w472) -> ()
    n276 = Wait (ms)(milliseconds to wait=u32 1000 ("等待时间（毫秒）")) -> ()  [unwired: 1 out]
    n277 = global read "氨氮断电保存全局变量.vi" "远程标样校准"() -> (w467:enum16{"标液1", "标液2", "标液3", "标液4"})
    n278 = global read "氨氮断电保存全局变量.vi" "远程校准量程"() -> (w466:enum16{"低量程", "高量程"})
    n279 = local write "远程标样校准"(w467) -> ()
    n280 = local write "远程校准量程"(w466) -> ()
  }
  n281 = while {
    tunnel: w27 -> [w511]
    tunnel: w26 -> [w510]
    tunnel: w25 -> [w509]
    tunnel: w24 -> [w508]
    tunnel: w23 -> [w507]
    tunnel: w13 -> [w506]
    tunnel: w18 -> [_]
    tunnel: w14 -> [w505]
    stop <- FALSE stop-if-true
    n282 = event shown="[16] \"设置\": 值改变" {
      selector: _ -> [_ _ _ _ _ _ _ _ _ _ _ _ _ _ _ _ _ _ _ _ _ _ _]
      dyn-events: _ -> [_ _ _ _ _ _ _ _ _ _ _ _ _ _ _ _ _ _ _ _ _ _ _]
      timeout: _ -> [_ _ _ _ _ _ _ _ _ _ _ _ _ _ _ _ _ _ _ _ _ _ _]
      tunnel: w511 -> [_ _ _ _ w539 _ w555 _ _ _ w573 _ _ w647 _ w669 _ _ _ _ _ _ _]
      tunnel: w510 -> [_ _ _ w517 _ _ _ _ _ _ _ _ _ _ _ _ w675 _ _ w698 w701 _ _]
      tunnel: w509 -> [_ _ _ w519 _ _ _ _ _ _ _ _ _ _ _ _ w677 _ _ w696 w703 w761 w768]
      tunnel: w508 -> [_ _ _ w518 _ _ _ _ _ _ _ _ _ _ _ _ w676 _ _ w697 w702 _ _]
      tunnel: w507 -> [_ _ _ w520 _ _ _ _ _ _ _ _ _ _ _ _ w678 _ _ w694 _ _ _]
      tunnel: w506 -> [_ _ _ _ _ _ _ _ _ _ _ _ _ _ _ _ w672 _ _ _ _ w759 _]
      tunnel: w505 -> [_ _ _ _ _ _ _ _ _ _ _ _ _ _ _ w664 _ _ _ _ _ _ _]
      tunnel: [_ _ _ w525 _ _ _ _ _ _ _ _ _ _ _ _ _ _ _ _ _ _ _] -> _
      event Timeout {
        n283 = event-data() -> ()  [unwired: 1 in, 3 out]
      }
      event "布尔": Mouse Down {
        n284 = event-data() -> ("CtlRef"=w514:refnum<vi>)  [unwired: 1 in, 5 out]
        n285 = property class="Bool (严格)"(reference=w514) -> ("Value"=w513:bool)  [unwired: 1 in, 2 out]
        n286 = case shown="真" w513 {
          frame False {
            n287 = call "密码键盘.vi"() -> ("NewNumber"=→"输入密码":dbl)  [unwired: 1 in]
          }
          frame True {
            n288 = local write "输入密码"(u32 0 ("输入密码")) -> ()
          }
        }
      }
      event "流程固件": Value Change {
        n289 = event-data() -> ()  [unwired: 1 in, 6 out]
        n290 = call "流程固件设置对话框.vi"() -> ()  [unwired: 12 in]
      }
      event "测量模式下拉列表", "量程下拉列表", "参数下拉列表": Value Change {
        n291 = event-data() -> ()  [unwired: 1 in, 6 out]
        n292 = property class="Enum (严格)"(reference=w519) -> ("Value"=w524:enum16{"总磷", "总氮", "氨氮"})  [unwired: 1 in, 2 out]
        n293 = property class="Enum (严格)"(reference=w518) -> ("Value"=w523:enum16{"水样测量", "零点核查", "跨度核查", "标样核查", "加标回收"})  [unwired: 1 in, 2 out]
        n294 = property class="Enum (严格)"(reference=w517) -> ("Value"=w522:enum16{"低量程", "高量程"})  [unwired: 1 in, 2 out]
        n295 = call "公式读取.vi"("量程"=w522, "测量模式"=w523, "测量参数"=w524) -> ("公式"=w521:cluster{"X^2":dbl, "X":dbl, "b":dbl})  [unwired: 7 in, 1 out]
        n296 = property class="Clust (严格)"(reference=w520, "Value"=w521) -> ()  [unwired: 1 in, 2 out]
        n297 = local read "测量模式下拉列表"() -> (w528:enum16{"水样测量", "零点核查", "跨度核查", "标样核查", "加标回收"})
        n298 = local read "量程下拉列表"() -> (w529:enum16{"低量程", "高量程"})
        n299 = local read "参数下拉列表"() -> (w527:enum16{"总磷", "总氮", "氨氮"})
        n300 = Bundle("参数下拉列表"=w527, "测量模式下拉列表"=w528, "量程下拉列表"=w529) -> (w526:T19)  [unwired: 1 in]
        n301 = property on="曲线模型" class="曲线模型 (严格)"("属性"=w526) -> (error out=w525:errorcluster)  [unwired: 2 in, 1 out]
      }
      event "串口设置": Value Change {
        n302 = event-data() -> ()  [unwired: 1 in, 6 out]
        n303 = global read "氨氮断电保存全局变量.vi" "VISA Resource"() -> (w536:refnum<visa-resource-name>)
        n304 = global read "氨氮断电保存全局变量.vi" "MB通信方式选择"() -> (w530:enum16{"串口", "TCP"})
        n305 = global read "氨氮断电保存全局变量.vi" "IP"() -> (w535:string)
        n306 = global read "氨氮断电保存全局变量.vi" "PORT"() -> (w534:string)
        n307 = call "串口配置.vi"("PORT"=w534, "IP"=w535, "MB通信方式选择"=w530, "请选择串口:"=w536) -> ("PORT 2"=w532:string, "IP 2"=w533:string, "确认 2"=w537:bool, "VISA资源名称 2"=w538:refnum<visa-resource-name>, "MB通信方式选择 2"=w531:enum16{"串口", "TCP"})  [unwired: 3 in]
        n308 = case shown="真" w537 {
          tunnel: w538 -> [_ w544]
          tunnel: w539 -> [_ w543]
          tunnel: w533 -> [_ w542]
          tunnel: w532 -> [_ w541]
          tunnel: w531 -> [_ w540]
          frame False {
          }
          frame True {
            n309 = flat-sequence {
              tunnel: w544 -> [w549]
              tunnel: w543 -> [w550]
              tunnel: w542 -> [w548]
              tunnel: w541 -> [w547]
              tunnel: w540 -> [w546]
              frame #0 {
                n310 = global write "氨氮断电保存全局变量.vi" "VISA Resource"(w549) -> ()
                n311 = global write "氨氮断电保存全局变量.vi" "IP"(w548) -> ()
                n312 = global write "氨氮断电保存全局变量.vi" "PORT"(w547) -> ()
                n313 = global write "氨氮断电保存全局变量.vi" "MB通信方式选择"(w546) -> ()
                n314 = Flush Queue(queue=w550) -> (queue out=w545:refnum<queue>)  [unwired: 1 in, 2 out]
                n315 = Enqueue Element(queue=w545, element=cluster{"命令":string, "data":variant} {"命令"="启用模块", "data"=variant} ("元素")) -> ()  [unwired: 2 in, 3 out]
              }
              frame #1 {
                n316 = call "配置文件保存.vi"() -> ()  [unwired: 11 in, 1 out]
              }
            }
          }
        }
      }
      event "远程校准量程", "远程标样校准": Value Change {
        n317 = event-data() -> ()  [unwired: 1 in, 6 out]
        n318 = flat-sequence {
          frame #0 {
            n319 = global write "氨氮断电保存全局变量.vi" "远程标样校准"("远程标样校准") -> ()
            n320 = global write "氨氮断电保存全局变量.vi" "远程校准量程"("远程校准量程") -> ()
          }
          frame #1 {
            n321 = call "配置文件保存.vi"() -> ()  [unwired: 11 in, 1 out]
          }
        }
      }
      event "模块启用": Value Change {
        n322 = event-data() -> ("OldVal"=w556:bool)  [unwired: 1 in, 5 out]
        n323 = Flush Queue(queue=w555) -> (queue out=w554:refnum<queue>)  [unwired: 1 in, 2 out]
        n324 = case shown="假" w556 {
          tunnel: w554 -> [w557 w559]
          frame False {
            n325 = Enqueue Element(queue=w557, element=cluster{"命令":string, "data":variant} {"命令"="停用模块", "data"=variant} ("元素")) -> ()  [unwired: 2 in, 3 out]
          }
          frame True {
            n326 = Enqueue Element(queue=w559, element=cluster{"命令":string, "data":variant} {"命令"="启用模块", "data"=variant} ("元素")) -> ()  [unwired: 2 in, 3 out]
          }
        }
      }
      event "流程路径": Value Change {
        n327 = event-data() -> ()  [unwired: 1 in, 6 out]
        n328 = flat-sequence {
          frame #0 {
            n329 = local read "流程路径"() -> (w561:path)
            n330 = global write "氨氮断电保存全局变量.vi" "流程路径"(w561) -> ()
          }
          frame #1 {
            n331 = call "配置文件保存.vi"() -> ()  [unwired: 11 in, 1 out]
          }
        }
      }
      event "公式一键写入": Value Change {
        n332 = event-data() -> ()  [unwired: 1 in, 6 out]
        n333 = local read "公式"() -> (w562:cluster{"X^2":dbl, "X":dbl, "b":dbl})
        n334 = call "公式复合写入.vi"("公式"=w562) -> ()  [unwired: 11 in]
      }
      event "曲线模型": Value Change {
        n335 = event-data() -> ()  [unwired: 1 in, 6 out]
        n336 = disable-structure shown="禁用" {
          frame Disabled {
            n337 = Unbundle By Name("曲线模型") -> ("X^2"=w565:dbl, "X"=w566:dbl, "B"=w567:dbl)
            n338 = Build Array(w565, w566, w567) -> (w564:dbl[])
            n339 = Array To Cluster(array=w564) -> (cluster=w563:cluster{"[0]":dbl, "[1]":dbl, "[2]":dbl})
            n340 = local write "公式"(w563) -> ()
          }
          frame Enabled {
          }
        }
      }
      event "校准按钮.校准1", "校准按钮.校准2", "校准按钮.校准3", "校准按钮.校准4", "校准按钮.校准5": Value Change {
        n341 = event-data() -> ("CtlRef"=w580:refnum<vi>)  [unwired: 1 in, 5 out]
        n342 = property class="Bool (严格)"(reference=w580) -> ("Label.Text"=w579:string)  [unwired: 1 in, 2 out]
        n343 = property on="曲线模型" class="曲线模型 (严格)"() -> ("浓度属性"=w576:T24)  [unwired: 2 in, 2 out]
        n344 = case shown="\"校准1\", 默认" w579 {
          tunnel: [w586 w589 w592 w595 w598] -> w572
          tunnel: [u16 1 ("校准点1-5") u16 2 ("校准点1-5") u16 3 ("校准点1-5") u16 4 ("校准点1-5") u16 5 ("校准点1-5")] -> w577
          tunnel: w576 -> [w587 w590 w593 w596 w599]
          frame "校准1", Default {
            n345 = Unbundle By Name(w587) -> ("标液浓度1"=w586:dbl)
          }
          frame "校准2" {
            n346 = Unbundle By Name(w590) -> ("标液浓度2"=w589:dbl)
          }
          frame "校准3" {
            n347 = Unbundle By Name(w593) -> ("标液浓度3"=w592:dbl)
          }
          frame "校准4" {
            n348 = Unbundle By Name(w596) -> ("标液浓度4"=w595:dbl)
          }
          frame "校准5" {
            n349 = Unbundle By Name(w599) -> ("标液浓度5"=w598:dbl)
          }
        }
        n350 = Not Equal To 0?(x=w572) -> (x != 0?=w571:bool)
        n351 = Bundle By Name(cluster=cluster{"校准？":bool, "校准点1-5":u16, "校准浓度":dbl} {"校准？"=FALSE, "校准点1-5"=0, "校准浓度"=0.0} ("校准输出"), "校准？"=TRUE, "校准点1-5"=w577, "校准浓度"=w572) -> (w575:cluster{"校准？":bool, "校准点1-5":u16, "校准浓度":dbl})
        n352 = global write "氨氮断电保存全局变量.vi" "校准输出"(w575) -> ()
        n353 = local read "量程下拉列表"() -> (w569:enum16{"低量程", "高量程"})
        n354 = case shown="假" w571 {
          tunnel: [cluster{"命令":string, "data":variant} {"命令"="启动", "data"=variant(cluster{"站号":u16, "控制命令":u16[]} {"站号"=3, "控制命令"=[2048, 256]})} ("元素") w583] -> w570
          tunnel: w569 -> [_ w582]
          frame False {
            # "校零"
          }
          frame True {
            # "校标"
            n355 = case shown="\"高量程\"" w582 {
              tunnel: [cluster{"命令":string, "data":variant} {"命令"="启动", "data"=variant(cluster{"站号":u16, "控制命令":u16[]} {"站号"=3, "控制命令"=[2304, 256]})} ("元素") cluster{"命令":string, "data":variant} {"命令"="启动", "data"=variant(cluster{"站号":u16, "控制命令":u16[]} {"站号"=3, "控制命令"=[2304, 257]})} ("元素")] -> w583
              frame "低量程", Default {
              }
              frame "高量程" {
              }
            }
          }
        }
        n356 = Enqueue Element(queue=w573, element=w570) -> ()  [unwired: 2 in, 3 out]
      }
      event "质控参数设置": Value Change {
        n357 = event-data() -> ()  [unwired: 1 in, 6 out]
        n358 = global read "氨氮断电保存全局变量.vi" "自动测试量程配置"() -> (w602:T25)
        n359 = global read "氨氮断电保存全局变量.vi" "质控参数设置"() -> (w603:T26)
        n360 = call "质控参数设置.vi"("自动测试量程配置"=w602, "质控参数设置"=w603) -> ("自动测试量程配置输出"=w601:T25, "输出簇"=w604:T27)  [unwired: 7 in]
        n361 = Unbundle By Name(w604) -> ("确定"=w605:bool)
        n362 = case shown="真" w605 {
          tunnel: w604 -> [_ w608]
          tunnel: w603 -> [_ w607]
          tunnel: w601 -> [_ w606]
          frame False {
          }
          frame True {
            n363 = flat-sequence {
              tunnel: w608 -> [w616]
              tunnel: w607 -> [w615]
              tunnel: w606 -> [w609]
              frame #0 {
                n364 = global write "氨氮断电保存全局变量.vi" "自动测试量程配置"(w609) -> ()
                n365 = Unbundle By Name(w616) -> ("跨度值"=w614:dbl, "零点标准液浓度"=w613:dbl, "跨度标准液浓度"=w612:dbl, "标准液标准浓度"=w611:dbl)
                n366 = Bundle By Name(cluster=w615, "跨度值"=w614, "零点标准液浓度"=w613, "跨度标准液浓度"=w612, "标准液标准浓度"=w611) -> (w610:T26)
                n367 = global write "氨氮断电保存全局变量.vi" "质控参数设置"(w610) -> ()
              }
              frame #1 {
                n368 = call "配置文件保存.vi"() -> ()  [unwired: 11 in, 1 out]
              }
            }
          }
        }
      }
      event "仪器参数设置": Value Change {
        n369 = event-data() -> ()  [unwired: 1 in, 6 out]
        n370 = global read "氨氮断电保存全局变量.vi" "氨氮仪器参数"() -> (w617:T28)
        n371 = call "仪器参数设置.vi"("氨氮仪器参数"=w617) -> ("仪器参数设置输出"=w618:T29)  [unwired: 10 in]
        n372 = Unbundle By Name(w618) -> ("确定"=w619:bool)
        n373 = case shown="真" w619 {
          tunnel: w618 -> [_ w621]
          tunnel: w617 -> [_ w620]
          frame False {
          }
          frame True {
            n374 = flat-sequence {
              tunnel: w621 -> [w637]
              tunnel: w620 -> [w636]
              frame #0 {
                n375 = Unbundle By Name(w637) -> ("测量量程"=w635:dbl, "测量精度"=w634:dbl, "测量间隔"=w633:dbl, "消解温度"=w632:dbl, "消解时长"=w630:dbl, "空白校准时间"=w629:timestamp, "曲线截距"=w628:dbl, "曲线斜率"=w627:dbl, "测量检出限"=w626:dbl, "测量信号值"=w625:dbl, "线性相关系数"=w624:dbl, "二次多项式系数"=w623:dbl, "标样校准时间"=w622:timestamp)
                n376 = Bundle By Name(cluster=w636, "测量量程"=w635, "测量精度"=w634, "测量间隔"=w633, "消解温度"=w632, "消解时长"=w630, "空白校准时间"=w629, "曲线截距"=w628, "曲线斜率"=w627, "测量检出限"=w626, "测量信号值"=w625, "线性相关系数"=w624, "二次多项式系数"=w623, "标样校准时间"=w622) -> (w631:T28)
                n377 = global write "氨氮断电保存全局变量.vi" "氨氮仪器参数"(w631) -> ()
              }
              frame #1 {
                n378 = call "配置文件保存.vi"() -> ()  [unwired: 11 in, 1 out]
              }
            }
          }
        }
      }
      event "手动启动": Value Change {
        n379 = event-data() -> ()  [unwired: 1 in, 6 out]
        n380 = call "氨氮启动参数对话框.vi"() -> ("标样浓度输出"=w639:dbl, "确认"=w646:bool, "元素"=w645:cluster{"命令":string, "data":variant})  [unwired: 9 in]
        n381 = case shown="真" w646 {
          tunnel: w647 -> [_ w662]
          tunnel: w645 -> [_ w661]
          frame False {
          }
          frame True {
            n382 = Enqueue Element(queue=w662, element=w661) -> ()  [unwired: 2 in, 3 out]
          }
        }
        n383 = Unbundle By Name(w645) -> ("data"=w643:variant)
        n384 = Variant To Data(type=cluster{"站号":u16, "控制命令":u16[]} {"站号"=0, "控制命令"=[]} ("输出簇"), Variant=w643) -> (data=w642:cluster{"站号":u16, "控制命令":u16[]})  [unwired: 1 in, 1 out]
        n385 = Unbundle By Name(w642) -> ("控制命令"=w641:u16[])
        n386 = Index Array(array=w641) -> (element=w640:u16)  [unwired: 1 in]
        n387 = Swap Bytes(anything=w640) -> (byte swapped=w638:u16)
        n388 = case shown="9" w638 {
          tunnel: w639 -> [_ w648 _ _]
          frame 0, Default {
          }
          frame 2 {
            # "标样核查"
            n389 = flat-sequence {
              tunnel: w648 -> [w649]
              frame #0 {
                n390 = global read "氨氮断电保存全局变量.vi" "质控参数设置"() -> (w651:T26)
                n391 = Bundle By Name(cluster=w651, "标准液标准浓度"=w649) -> (w650:T26)
                n392 = global write "氨氮断电保存全局变量.vi" "质控参数设置"(w650) -> ()
              }
              frame #1 {
                n393 = call "配置文件保存.vi"() -> ()  [unwired: 11 in, 1 out]
              }
            }
          }
          frame 8 {
            # "空白校准"
            n394 = property on="校准1" class="Bool (严格)"("Val(Sgnl)"=TRUE ("值(信号)")) -> ()  [unwired: 2 in, 2 out]
            n395 = property on="量程下拉列表" class="Enum (严格)"("Val(Sgnl)"=enum16{"低量程", "高量程"}."低量程" ("值(信号)")) -> ()  [unwired: 2 in, 2 out]
          }
          frame 9 {
            # "标样校准"
            n396 = local read "远程标样校准"() -> (w656:enum16{"标液1", "标液2", "标液3", "标液4"})
            n397 = case shown="\"标液1\", 默认" w656 {
              tunnel: TRUE ("值(信号)") -> [w657 w658 w659 w660]
              frame "标液1", Default {
                n398 = property on="校准2" class="Bool (严格)"("Val(Sgnl)"=w657) -> ()  [unwired: 2 in, 2 out]
              }
              frame "标液2" {
                n399 = property on="校准3" class="Bool (严格)"("Val(Sgnl)"=w658) -> ()  [unwired: 2 in, 2 out]
              }
              frame "标液3" {
                n400 = property on="校准4" class="Bool (严格)"("Val(Sgnl)"=w659) -> ()  [unwired: 2 in, 2 out]
              }
              frame "标液4" {
                n401 = property on="校准5" class="Bool (严格)"("Val(Sgnl)"=w660) -> ()  [unwired: 2 in, 2 out]
              }
            }
            n402 = local read "远程校准量程"() -> (w654:enum16{"低量程", "高量程"})
            n403 = property on="量程下拉列表" class="Enum (严格)"("Val(Sgnl)"=w654) -> ()  [unwired: 2 in, 2 out]
          }
        }
      }
      event "单步测试": Value Change {
        n404 = event-data() -> ()  [unwired: 1 in, 6 out]
        n405 = call "氨氮单步调试对话框.vi"() -> ()  [unwired: 12 in]
      }
      event "停止": Value Change {
        n406 = event-data() -> ()  [unwired: 1 in, 6 out]
        n407 = Cancel Notification(0:w664) -> (8:w665:refnum<notifier>)  [unwired: 1 in, 2 out]
        n408 = Enqueue Element(queue=w669, element=cluster{"命令":string, "data":variant} {"命令"="启动", "data"=variant(cluster{"站号":u16, "控制命令输出":u16[]} {"站号"=1, "控制命令输出"=[2816]})} ("元素")) -> (queue out=w666:refnum<queue>)  [unwired: 2 in, 2 out]
        n409 = Send Notification(notification=TRUE ("通知"), notifier=w665) -> ()  [unwired: 1 in, 2 out]
        n410 = Enqueue Element(queue=w666, element=cluster{"命令":string, "data":variant} {"命令"="启动", "data"=variant(cluster{"站号":u16, "控制命令输出":u16[]} {"站号"=2, "控制命令输出"=[2816]})} ("元素")) -> ()  [unwired: 2 in, 3 out]
      }
      event "设置": Value Change {
        n411 = event-data() -> ()  [unwired: 1 in, 6 out]
        n412 = property class="Enum (严格)"(reference=w677) -> (reference out=w671:refnum<vi>, "Value"=w682:enum16{"总磷", "总氮", "氨氮"})  [unwired: 1 in, 1 out]
        n413 = property class="Enum (严格)"(reference=w676) -> ("Value"=w681:enum16{"水样测量", "零点核查", "跨度核查", "标样核查", "加标回收"})  [unwired: 1 in, 2 out]
        n414 = property class="Enum (严格)"(reference=w675) -> ("Value"=w680:enum16{"低量程", "高量程"})  [unwired: 1 in, 2 out]
        n415 = property on="窗格" class="Pane"("Origin"=T7 {"Horizontal"=0, "Vertical"=628} ("原点")) -> ()  [unwired: 2 in, 2 out]
        n416 = call "公式读取.vi"("量程"=w680, "测量模式"=w681, "测量参数"=w682) -> ("error out"=w670:errorcluster, "公式"=w679:cluster{"X^2":dbl, "X":dbl, "b":dbl})  [unwired: 7 in]
        n417 = property class="Clust (严格)"(reference=w678, "Value"=w679) -> ()  [unwired: 1 in, 2 out]
        n418 = property class="Enum (严格)"(reference=w671) -> ("Value"=w674:enum16{"总磷", "总氮", "氨氮"})  [unwired: 1 in, 2 out]
        n419 = call "量程读取.vi"("error in (no error)"=w670, "测量参数"=w674) -> ("量程参数读取"=w673:T30)  [unwired: 8 in, 1 out]
        n420 = property class="Clust (严格)"(reference=w672, "Value"=w673) -> ()  [unwired: 1 in, 2 out]
      }
      event "返回": Value Change {
        n421 = event-data() -> ()  [unwired: 1 in, 6 out]
        n422 = property on="窗格" class="Pane"("Origin"=T7 {"Horizontal"=0, "Vertical"=0} ("原点")) -> ()  [unwired: 2 in, 2 out]
      }
      event "公式.X^2", "公式.X", "公式.b", "量程参数读取写入.测量精度", "量程参数读取写入.检出限", "量程参数读取写入.上限", "量程参数读取写入.下限", "量程参数读取写入.阈值(低->高)", "量程参数读取写入.(高->低)", "量程参数读取写入.稀释度": Mouse Down {
        n423 = event-data() -> ("CtlRef"=w688:refnum<vi>)  [unwired: 1 in, 5 out]
        n424 = property class="DigNum (严格)"(reference=w688) -> (reference out=w686:refnum<vi>, "Value"=w687:dbl)  [unwired: 1 in, 1 out]
        n425 = call "数字键盘.vi"("OldNumber"=w687) -> ("NewNumber"=w685:dbl)
        n426 = property class="DigNum (严格)"(reference=w686, "Val(Sgnl)"=w685) -> ()  [unwired: 1 in, 2 out]
      }
      event "读公式": Value Change {
        n427 = event-data() -> ()  [unwired: 1 in, 6 out]
        n428 = property class="Enum (严格)"(reference=w696) -> ("Value"=w695:enum16{"总磷", "总氮", "氨氮"})  [unwired: 1 in, 2 out]
        n429 = property class="Enum (严格)"(reference=w697) -> ("Value"=w692:enum16{"水样测量", "零点核查", "跨度核查", "标样核查", "加标回收"})  [unwired: 1 in, 2 out]
        n430 = property class="Enum (严格)"(reference=w698) -> ("Value"=w691:enum16{"低量程", "高量程"})  [unwired: 1 in, 2 out]
        n431 = call "公式读取.vi"("量程"=w691, "测量模式"=w692, "测量参数"=w695) -> ("error out"=w689:errorcluster, "公式"=w690:cluster{"X^2":dbl, "X":dbl, "b":dbl})  [unwired: 7 in]
        n432 = property class="Clust (严格)"(reference=w694, "Value"=w690) -> ()  [unwired: 1 in, 2 out]
        n433 = case shown="无错误" w689 {
          tunnel: ["读取成功" ("消息") "读取失败" ("消息")] -> w693
          frame No Error {
          }
          frame Error {
          }
        }
        n434 = One Button Dialog(message=w693) -> ()  [unwired: 1 in, 1 out]
      }
      event "写公式": Value Change {
        n435 = event-data() -> ()  [unwired: 1 in, 6 out]
        n436 = call <vilib>:"Three Button Dialog.vi"("Allow user to close window? (TRUE)"=FALSE, "Center Button Text (\"No\")"="一键写入所有模式公式" ("F按钮名称（“取消”）"), "Left Button Text (\"Yes\")"="写入当前模式公式" ("T按钮名称（“确定”）"), "message"="即将将左侧拟合公式写入仪器\n请选择写入当前模式还是一键写入所有模式！" ("消息")) -> ("Which Button?"=w704:T31)  [unwired: 7 in]
        n437 = case shown="\"Left Button\"" w704 {
          tunnel: w703 -> [w715 w749 _ _]
          tunnel: w702 -> [w714 w748 _ _]
          tunnel: w701 -> [w713 w747 _ _]
          frame "Left Button" {
            n438 = local read "曲线模型"() -> (w720:cluster{"X^2":dbl, "X":dbl, "B":dbl, "r^2":dbl})
            n439 = Unbundle By Name(w720) -> ("X^2"=w718:dbl, "X"=w717:dbl, "B"=w716:dbl)
            n440 = Build Array(w718, w717, w716) -> (w719:dbl[])
            n441 = Array To Cluster(array=w719) -> (cluster=w712:cluster{"[0]":dbl, "[1]":dbl, "[2]":dbl})
            n442 = call "公式写入.vi"("公式"=w712, "量程"="量程下拉列表", "测量模式"="测量模式下拉列表", "测量参数"="参数下拉列表") -> ("error out"=w724:errorcluster)  [unwired: 7 in]
            n443 = local write "公式"(w712) -> ()
            n444 = case shown="无错误" w724 {
              tunnel: ["写入成功" ("消息") "写入失败" ("消息")] -> w725
              tunnel: "测量模式下拉列表" -> [w734 _]
              tunnel: "量程下拉列表" -> [w733 _]
              tunnel: w712 -> [w729 _]
              frame No Error {
                n445 = Unbundle By Name(w729) -> ("[0]"=w728:dbl, "[1]"=w727:dbl, "[2]"=w726:dbl)
                n446 = Equal?(x=w734, y=enum16{"水样测量", "零点核查", "跨度核查", "标样核查", "加标回收"}."水样测量") -> (x = y?=w732:bool)
                n447 = Equal?(x=w733, y=enum16{"低量程", "高量程"}."低量程") -> (x = y?=w731:bool)
                n448 = Compound Arithmetic op=AND ("复合运算")(w732, w731) -> (w730:bool)
                n449 = case shown="真" w730 {
                  tunnel: w728 -> [_ w740]
                  tunnel: w727 -> [_ w739]
                  tunnel: w726 -> [_ w738]
                  frame False {
                  }
                  frame True {
                    n450 = global read "氨氮断电保存全局变量.vi" "氨氮仪器参数"() -> (w741:T28)
                    n451 = Bundle By Name(cluster=w741, "曲线截距"=w738, "曲线斜率"=w739, "二次多项式系数"=w740) -> (w742:T28)
                    n452 = global write "氨氮断电保存全局变量.vi" "氨氮仪器参数"(w742) -> ()
                  }
                }
              }
              frame Error {
              }
            }
            n453 = call "公式发生改变存储 (子VI).vi"("公式"=w712, "量程下拉列表输入"=w713, "测量模式下拉列表输入"=w714, "参数"=w715) -> ()  [unwired: 8 in]
            n454 = control-ref of="量程下拉列表"() -> (w710:refnum<vi>)
            n455 = control-ref of="曲线模型"() -> (w711:refnum<vi>)
            n456 = call "生成校准信息.vi"("table输入"="氨氮", "量程下拉列表"=w710, "曲线模型"=w711) -> ()  [unwired: 9 in]
            n457 = One Button Dialog(message=w725) -> ()  [unwired: 1 in, 1 out]
          }
          frame "Center Button" {
            n458 = local read "曲线模型"() -> (w755:cluster{"X^2":dbl, "X":dbl, "B":dbl, "r^2":dbl})
            n459 = Unbundle By Name(w755) -> ("X^2"=w753:dbl, "X"=w752:dbl, "B"=w751:dbl)
            n460 = Build Array(w753, w752, w751) -> (w754:dbl[])
            n461 = Array To Cluster(array=w754) -> (cluster=w750:cluster{"[0]":dbl, "[1]":dbl, "[2]":dbl})
            n462 = local write "公式"(w750) -> ()
            n463 = call "公式发生改变存储 (子VI).vi"("公式"=w750, "量程下拉列表输入"=w747, "测量模式下拉列表输入"=w748, "参数"=w749) -> ()  [unwired: 8 in]
            n464 = call "公式复合写入.vi"("公式"=w750) -> ()  [unwired: 11 in]
            n465 = control-ref of="量程下拉列表"() -> (w745:refnum<vi>)
            n466 = control-ref of="曲线模型"() -> (w746:refnum<vi>)
            n467 = call "生成校准信息.vi"("table输入"="氨氮", "量程下拉列表"=w745, "曲线模型"=w746) -> ()  [unwired: 9 in]
          }
          frame "Right Button", Default {
          }
          frame "Window Close" {
          }
        }
      }
      event "量程切换阈值读取": Value Change {
        n468 = event-data() -> ()  [unwired: 1 in, 6 out]
        n469 = property class="Enum (严格)"(reference=w761) -> ("Value"=w760:enum16{"总磷", "总氮", "氨氮"})  [unwired: 1 in, 2 out]
        n470 = call "量程读取.vi"("测量参数"=w760) -> ("error out"=w756:errorcluster, "量程参数读取"=w758:T30)  [unwired: 9 in]
        n471 = property class="Clust (严格)"(reference=w759, "Value"=w758) -> ()  [unwired: 1 in, 2 out]
        n472 = case shown="错误" w756 {
          tunnel: ["读取成功" ("消息") "读取失败" ("消息")] -> w757
          frame No Error {
          }
          frame Error {
          }
        }
        n473 = One Button Dialog(message=w757) -> ()  [unwired: 1 in, 1 out]
      }
      event "量程切换阈值写入": Value Change {
        n474 = event-data() -> ()  [unwired: 1 in, 6 out]
        n475 = property class="Enum (严格)"(reference=w768) -> ("Value"=w767:enum16{"总磷", "总氮", "氨氮"})  [unwired: 1 in, 2 out]
        n476 = call "量程写入.vi"("量程参数写入"="量程参数读取写入", "测量参数"=w767) -> ("error out"=w765:errorcluster)  [unwired: 8 in]
        n477 = case shown="无错误" w765 {
          tunnel: ["写入成功" ("消息") "写入失败" ("消息")] -> w766
          frame No Error {
          }
          frame Error {
          }
        }
        n478 = One Button Dialog(message=w766) -> ()  [unwired: 1 in, 1 out]
      }
    }
  }
  n479 = while {
    tunnel: [w778] -> _
    shift-right: [w776] -> _
    shift-left: w6 -> [w775]
    tunnel: w7 -> [w772]
    stop <- FALSE stop-if-true
    n480 = global read "VAR氨氮全局变量.vi" "配置文件 path"() -> (w771:path)
    n481 = Read from Text File(file (use dialog)=w771, error in=w772) -> (text=w776:string, error out=w773:errorcluster)  [unwired: 2 in, 2 out]
    n482 = Not Equal?(x=w776, y=w775) -> (x != y?=w774:bool)
    n483 = case shown="真" w774 {
      tunnel: [w780 w784] -> w778
      tunnel: w771 -> [_ w783]
      tunnel: w773 -> [w780 w782]
      frame False {
      }
      frame True {
        # "文件发生改变进行更新"
        n484 = call <vilib>:"Open Config Data.vi"("error in (no error)"=w782, "configuration file path"=w783) -> ("error out"=w788:errorcluster, "refnum"=w787:T16)  [unwired: 7 in, 1 out]
        n485 = vi-ref "氨氮断电保存全局变量.vi"() -> (w781:refnum<vi>)
        n486 = call <userlib>:"Read Panel from INI__ogtk.vi"("error in (no error)"=w788, "VI ref"=w781, "refnum"=w787) -> ("error out"=w786:errorcluster, "refnum out"=w785:T16)  [unwired: 7 in]
        n487 = call <vilib>:"Close Config Data.vi"("error in (no error)"=w786, "refnum"=w785) -> ("error out"=w784:errorcluster)  [unwired: 8 in, 1 out]
      }
    }
    n488 = Wait (ms)(milliseconds to wait=u32 1000 ("等待时间（毫秒）")) -> ()  [unwired: 1 out]
  }
